vi "ViewEye.vi"(5 "new file path":path) -> ()   [LabVIEW 2022 SP3]
uses:
  -ReadEye/ScaleMethod.ctl
  <vilib>/Utility/miscctls.llb/LVPointDoubleTypeDef.ctl
  <vilib>/Utility/miscctls.llb/LVRectTypeDef.ctl
  <vilib>/Utility/miscctls.llb/LVOffsetAndMultiplierTypeDef.ctl
  <vilib>/Utility/miscctls.llb/LVBoundsTypeDef.ctl
  <vilib>/Analysis/baseanly.llb/Mean (DBL).vi
  <vilib>/Analysis/5stat.llb/RMS (DBL).vi
  <vilib>/Analysis/4window.llb/Chebyshev Window (DBL).vi
  <vilib>/Analysis/2dsp.llb/Zero Padder (DBL).vi
  <vilib>/Utility/file.llb/Write Delimited Spreadsheet (DBL).vi
  <vilib>/Utility/file.llb/Write Delimited Spreadsheet (string).vi
  <vilib>/Utility/file.llb/Read Delimited Spreadsheet (I64).vi
  <vilib>/Analysis/NI_AALPro.lvlib
  <vilib>/Analysis/NI_AALBase.lvlib
  <vilib>/ptbypt/NI_PtbyPt.lvlib
  <vilib>/gmath/NI_Gmath.lvlib
  <vilib>/Analysis/NI_AAL_SigProc.lvlib
panel:
  in  "Ref data":path=path "C:/WINDOWS/DESKTOP/rri.eye"
  in  "y":dbl(slide) scale=-2.0..2.0
  in  "RMS Save":bool
  in  "Boolean":bool
  in  "Flip Y":bool
  in  "Flip X":bool
  in  "Fill":bool
  in  "1-to-1":bool
  out "File Name":string
  in  "previously\nscanned":string
  in  "Keeper?":bool
  out "Scan Info":T1
  in  "File Ext":string="*.eye"
  out "Sound Speed":i16=1485
  in  "One Way":bool
  in  "Prev File":bool
  in  "Scale":bool=TRUE
  in  "Type of Mean":u16(ring) items=["Mean from lines", "Mean just lines", "Poly Mean", "No mean", "Filter"]
  in  "Filter Prams":T2={"low cutoff"=5, "order"=81, "high cutoff"=65}
  out "Raw data":dbl[][](graph)
  in  "Retro Parse":bool
  in  "Avg Spec":bool
  in  "Tab Control":T3(tab)
  in  "dB scale":u16(ring)=1 items=["Absolute", "Zero Ref"]
  in  "Vert Scale":u16(ring)=1 items=["Binary", "Dig Voltage", "Abs Voltage", "RF File Att Pram"]
  in  "Save RF":bool
  out "Blow up of blue Line":dbl[][](graph)
  out "Spectrum":T4(graph)
  in  "FFT size for":u16(ring)=9 items=["next 2^n", "8", "16", "32", "64", "128", "256", "512", "1024", "2048", "4096", "8192", "16384"]
  in  "Save Spectra?":bool
  out "blue win":dbl[](array[numeric])
  in  "Fit band":T5 {"center freq" format="%.2f"; "stop freq" format="%.2f"; "start" format="%.2f"}
  out "max doppler velocity mm/s":dbl
  in  "Drop freq coumn?":bool
  in  "Slide":cluster{dbl, dbl}(slide)={0.0, -50.63291139240506} scale=-80.0..100.0
  out "dB":dbl[][](graph)
  in  "STFT size":u16(ring)=9 items=["next 2^n", "8", "16", "32", "64", "128", "256", "512", "1024", "2048", "4096", "8192", "16384"]
  in  "Window":u32(ring)=2 items=["Rectangle"=0, "Hanning"=1, "Hamming"=2, "Blackman-Harris"=3, "Exact Blackman"=4, "Blackman"=5, "Flat Top"=6, "4 Term B-Harris "=7, "7 Term B-Harris"=8, "Low Sidelobe"=9, "Blackman Nuttall"=11, "Triangle"=30, "Gaussian"=62]
  out "mean 2":dbl format="%0.2f"
  out "mean":dbl format="%0.2f"
  out "Waveform Graph 2":dbl[](graph)
  out "Waveform Graph":dbl[](graph)
  in  "Spectro BMP":bool
  in  "Shift":sgl
  out "max value":sgl
  out "Time step (mics)":dbl
  in  "Spectrum?":bool
  out "Spectro fig":dbl[][](graph)
  in  "step size":i32=4 min=0
  in  "window pts":i32=64 min=0
  in  "Save Chirp":bool
  out "Match Data":dbl[][](graph)
  out "Chirp Temp":dbl[][](array[numeric])
  in  "Match Filter":bool
  in  "Add Lines":u16=1
  out "Axis scaling Params":T6 {"Y high" format="%.2f"; "Y low" format="%.2f"; "X left" format="%.2f"; "X right" format="%.2f"}
  out "inc y (mm)":dbl format="%.3f"
  out "inc x (mm)":dbl format="%.3f"
  in  "Reduce x data factor":i32=1
  in  "Pixels in y":i16=2500
  in  "Pixels in x":i16=256
  in  "Save BMP?":bool
  in  "Create Sector":bool
  out "Sector as data array":dbl[][](graph)
  out "cursor":dbl
  in  "Smooth factor":i32=1
  out "XY Graph":T7(graph)
  in  "Histo":bool
  in  "sub thresh":dbl=25.0
  in  "Contrast Batch":bool
  out "Therapy amplitude (mV)":sgl min=50 max=1000 format="%.2f"
  out "time trace":dbl[][](graph)
  out "Sepctra":cluster{i32, "df":dbl, dbl[][]}(graph)
  in  "Contrast Spec":bool
  out "Hit frac":dbl
  out "?":cluster{dbl[], "Best Linear Fit":dbl[]}[](graph)
  out "histogram":T7(graph)
  in  "Center Line SNR":bool
  out "Peaks":dbl[](graph)
  in  "save lateral?":bool
  out "Wire Locations RF pts":dbl[](array[numeric]) format="%0.2f"
  in  "Lateral beam":bool
  out "Wire Locations mm":dbl[](array[numeric]) format="%0.2f"
  out "lat beams":dbl[][](graph)
  in  "Threshold":i32=5000
  in  "width":i32=10
  out "SNRs":dbl[](array[numeric])
  in  "Wires":i32=13
  in  "Center index":i32
  out "Scan Line Peak":dbl[](array[numeric]) format="%0.2f"
  out "Beamwidths":sgl[](array[numeric])
  in  "initial Skip index":i32=100
  in  "Heart Trig":bool
  out "Smooth dat":dbl(graph)
  out "Avg Env image":dbl[][](graph)
  out "Overlay":dbl[][](graph)
  in  "AS Med Fil":i32=20
  in  "Edge Thresh":i32=20
  in  "Thresh Median Lngth":i32=10
  in  "direction":enum16{"either", "minus-plus", "plus-minus"}(ring)=enum."minus-plus"
  in  "neg cross":dbl=-3.0
  in  "Ebedded EKG":bool
  out "EKG":i16[][](graph)
  in  "EKG Gate":u16(ring) items=["Retro EKG", "Retro IQ"]
  out "dB 2":dbl[][](graph)
  out "Raw data 2":dbl[][](graph)
  in  "medians":i32=-1
  in  "left rank":i32=2
  in  "Log noise window":bool
  in  "Log":bool
  in  "CNR?":bool
  in  "Save RMS":bool
  out "Waveform Graph 3":dbl[](graph)
  in  "Save RF in window":bool
  in  "row to show":i32
  out "RMS dB BG":dbl format="%#.3g"
  out "CNR":dbl
  out "RMS flow dB":dbl format="%#.3g"
  out "dB CBR":dbl format="%#.3g"
  out "Spectrum 2":dbl[][](graph)
  out "RMS noise dB":dbl format="%#.3g"
  out "pk dB":dbl format="%#.2f"
  out "Pts  flow":i32
  out "Pts BG":i32
  out "Values":T8
  in  "ROI (mm)":T9={"X"=10.0, "Y"=10.0}
  in  "Fix Window CNR":bool
  in  "Delete File":bool
  in  "Whole Image":bool
  in  "Syn Focus":bool
  in  "Eye to BMP":bool
  in  "View Pics":bool
  in  "Alter Header":bool
  in  "Next File in Dir?":bool
  out "RF Lines":i32
  out "RF Window Pts":i32
  in  "ExitSendCmd":bool
  in  "Display mode":T10=enum."Log Grey Scale"
  out "DynRange":dbl format="%#.2f"
  out "RMS noise":dbl format="%#.3g"
  in  "Add Switch Noise?":bool
  in  "Axis scaling":bool
  in  "View Header?":bool
  in  "Header format":u16(ring) items=["Riverside Format", "Ron Linear", "GE Bin"]
  # "© 2000-2013 Riverside Research Institute"
  # "Ignore if not using a sector scan"
  # "Character to add to header"
  # "Note columns of the raw data have been inverted\nand the resulting matrix has been transposed to form\nthe sector image. Data reduced from raw form"
  # "Crop sides with yellow line"
  # "Use mm scale."
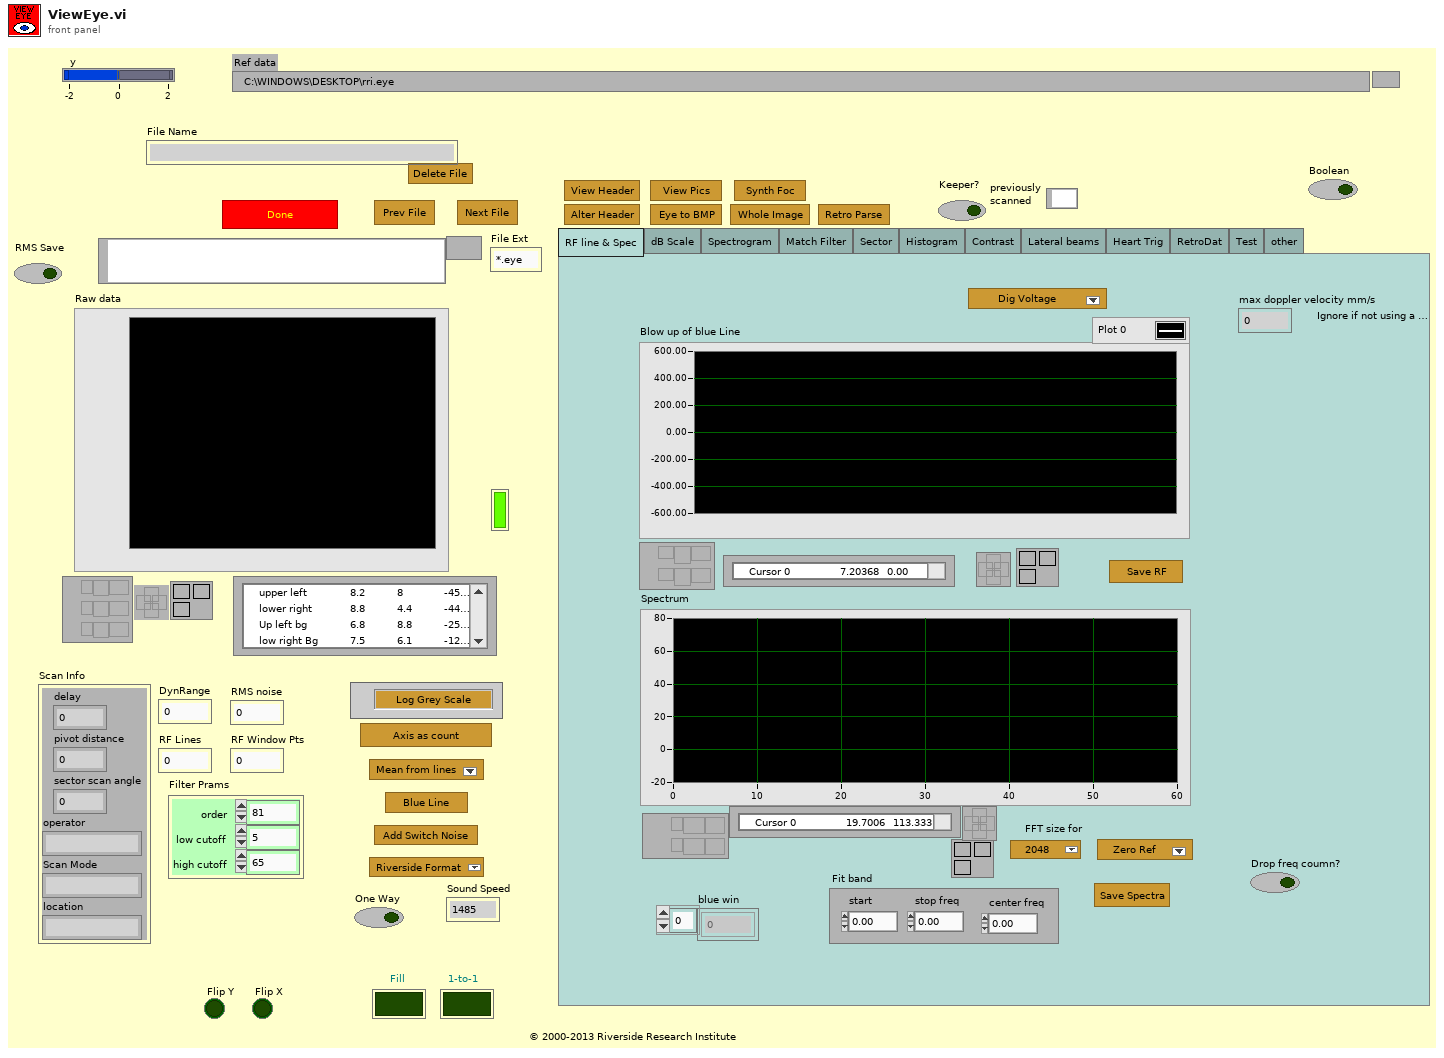
[diagram p1: front panel]
types:
  T1 = cluster{"delay":sgl, "pivot distance":sgl, "sector scan angle":sgl, "operator":string, "Scan Mode":string, "location":string}
  T2 = cluster{"low cutoff":i32, "order":i32, "high cutoff":i32}
  T3 = enum32{"RF line & Spec", "dB Scale", "Spectrogram", "Match Filter", "Sector", "Histogram", "Contrast", "Lateral beams", "Heart Trig", "RetroDat", "Test", "other"}
  T4 = cluster{"fo of fit":dbl, "df (MHz)":dbl, "Best Linear Fit":dbl[]}[]
  T5 = cluster{"start":dbl, "stop freq":dbl, "center freq":dbl}
  T6 = cluster{"X right":dbl, "X left":dbl, "Y low":dbl, "Y high":dbl}
  T7 = cluster{"X Values":dbl[], "Histogram: h(x)":i32[]}
  T8 = cluster{"mean":dbl, "variance":dbl, "mean":dbl, "variance":dbl}
  T9 = typedef "LVPointDoubleTypeDef.ctl" = cluster{"X":dbl, "Y":dbl}
  T10 = typedef "ScaleMethod.ctl" = enum16{"Linear Abs Grey", "Log Grey Scale", "Linear Color Scale", "dB Scale", "Verasonics Doppler"}
  T11 = typedef "LVRectTypeDef.ctl" = cluster{"Left":i16, "Top":i16, "Right":i16, "Bottom":i16}
  T12 = typedef "LVBoundsTypeDef.ctl" = cluster{"Width":u32, "Height":u32}
  T13 = cluster{"header info":cluster{"Header":string, "Head length":i16}, "A/D info":cluster{"# rf points per line":u16, "# lines per scan":u16, "sample rate MHz":u16, "# A/D bits":i16, "# bytes per A/D":u16, "TGC Flag":u16, "A/D Type":string}, "Tranducer Info":cluster{"bandwidth":sgl, "center freq":sgl, "start freq":sgl, "ID":i32}, "Scan Info":cluster{"delay":sgl, "pivot distance":sgl, "sector scan angle":sgl, "operator":string, "Scan Mode":string, "location":string}, "Time/Date Info":cluster{"date":string, "time":string}, "RF Info":cluster{"RF file name":string, "RF file att":string, "RF cal file name":string, "RF cal file att":string}, "Patient Info":cluster{"ID":string, "extended ID":string, "age":u16, "sex":string, "previously\nscanned":string, "PSA":sgl, "LOS":u8, "Ethnicty 2":u8, "Race":u8}, "Tissue Type":cluster{"organ":i16, "disease type":i16, "disease location":i16, "IQ_pts":u16, "RcvBuffer":u8, "RcvFrame":i16, "IQBuff":u8, "IQFrame":u16, "IQPage":u8}, "Votage scaling":cluster{"Digitizer (dB)":sgl, "Gain (dB)":sgl, "Atten (dB)":sgl}, "Comment":string, "Misc Items":cluster{"avg num":i16, "c speed":i16, "DivideBy":i16, "XMIT CHS":u8, "RCV CHS":u8, "Tx angle":u8}, "Therapy Parameters":cluster{"Theraputic Freq (MHz)":sgl, "Time on (s)":sgl, "Therapy amplitude (mV)":sgl, "Lines Before":u16, "Lines After":u16}, "Scan Settings":cluster{"Energy (microJ)":u8, "Damping (In Ohm)":u8, "HP Filt(KHz) ":u8, "LP Filt (MHz)":u8, "Gain (db)":u8, "prf (kHz)":sgl, "Distance between\nscan lines (mm)":u16, "Distance between\nscan planes (mm)":u16, "prf (kHz) 2":sgl, "prf (kHz) 3":sgl}, "Compression Parameters":cluster{"F1 (MHz)":sgl, "F2 (MHz)":sgl, "% taper":sgl, "duration":sgl}, "Patient Info Xtra":cluster{"First Name":string, "Last Name":string, "Notes":string}, "Boolean1":cluster{bool, bool, bool, bool, bool, bool, bool, bool, bool, bool, bool, bool, bool, bool, bool, bool, bool, bool, bool, bool, bool, bool}, "Boolean2":cluster{bool, bool, bool, bool, bool, bool, bool, bool, bool, bool, bool, bool, bool, bool, bool, bool, bool, bool, bool, bool, bool, bool, bool, bool, bool, bool, bool, bool, bool, bool, bool, bool, bool, bool, bool}, "Boolean3":cluster{bool, bool, bool, bool, bool, bool, bool, bool, bool, bool, bool, bool, bool, bool, bool, bool, bool, bool, bool, bool, bool, bool}}
  T14 = cluster{bool, bool, bool, bool, bool, bool, bool, bool, bool, bool, bool, bool, bool, bool, bool, bool, bool, bool, bool, bool, bool, bool}
  T15 = cluster{bool, bool, bool, bool, bool, bool, bool, bool, bool, bool, bool, bool, bool, bool, bool, bool, bool, bool, bool, bool, bool, bool, bool, bool, bool, bool, bool, bool, bool, bool, bool, bool, bool, bool, bool}
  T16 = enum16{"big-endian, network order", "native, host order", "little-endian"}
  T17 = typedef "Header.ctl" = cluster{"header info":cluster{"Header":string, "Head length":i16}, "A/D info":cluster{"# rf points per line":u16, "# lines per scan":u16, "sample rate MHz":u16, "# A/D bits":i16, "# bytes per A/D":u16, "TGC Flag":u16, "A/D Type":string}, "Tranducer Info":cluster{"bandwidth":sgl, "center freq":sgl, "start freq":sgl, "ID":i32}, "Scan Info":cluster{"delay":sgl, "pivot distance":sgl, "sector scan angle":sgl, "operator":string, "Scan Mode":string, "location":string}, "Time/Date Info":cluster{"date":string, "time":string}, "RF Info":cluster{"RF file name":string, "RF file att":string, "RF cal file name":string, "RF cal file att":string}, "Patient Info":cluster{"ID":string, "extended ID":string, "age":u16, "sex":string, "previously\nscanned":string, "PSA":sgl, "LOS":u8, "Ethnicty 2":u8, "Race":u8}, "Tissue Type":cluster{"organ":i16, "disease type":i16, "disease location":i16, "IQ_pts":u16, "RcvBuffer":u8, "RcvFrame":u16, "IQBuff":u8, "IQFrame":u16, "IQPage":u8}, "Votage scaling":cluster{"Digitizer (dB)":sgl, "Gain (dB)":sgl, "Atten (dB)":sgl}, "Comment":string, "Misc Info":cluster{"avg num":u16, "c speed":i16, "Div By or SF zones":i16, "XMIT CHS":u8, "RCV CHS":u8, "Xmit angle":sgl}, "Therapy Parameters":cluster{"Theraputic Freq (MHz)":sgl, "Time on (s)":sgl, "Therapy amplitude (mV)":sgl, "Lines Before":u16, "Lines After":u16}, "Scan Settings":cluster{"Energy (uJ or V)":u8, "Damp (Ohm) or Fc":u8, "HP Filt (KHz)":u8, "LP Filt (MHz)":u8, "Gain (db)":u8, "prf (kHz)":sgl, "Distance between\nscan lines (um)":u16, "Distance between\nscan planes (um)":u16, "Scan line gap (um)":sgl, "Scan plane gap (um)":sgl}, "Compression Parameters":cluster{"F1 (MHz)":sgl, "F2 (MHz)":sgl, "% taper":sgl, "duration":sgl}, "Patient Info Xtra":cluster{"First Name":string, "Last Name":string, "Notes":string}, "ROI Box":u16[]}
  T18 = cluster{"fo of fit":dbl, "df (MHz)":dbl, "Best Linear Fit":dbl[]}
  T19 = typedef "LVOffsetAndMultiplierTypeDef.ctl" = cluster{"Offset":dbl, "Multiplier":dbl}
  T20 = typedef "imagedata.ctl" = cluster{"image type":i32, "image depth":i32, "image":u8[], "mask":u8[], "colors":u32[], "Rectangle":cluster{"left":i16, "top":i16, "right":i16, "bottom":i16}}
  T21 = typedef "eventvkey.ctl" = enum16{"ASCII", "Enter", "Return", "Shift", "Ctrl", "Alt", "Cmd", "Opt", "Caps", "NumLock", "Clear", "Break", "Up", "Down", "Left", "Right", "Insert", "Delete", "Home", "End", "PageUp", "PageDown", "Escape", "Help", "Pause", "ScrollLock", "F1", "F2", "F3", "F4", "F5", "F6", "F7", "F8", "F9", "F10", "F11", "F12", "F13", "F14", "F15", "F16", "F17", "F18", "F19", "F20", "F21", "F22", "F23", "F24", "Play", "VolumeUp", "VolumeDown", "Mute", "Two Byte Char"}
  T22 = cluster{"Energy (microJ)":u8, "Damping (In Ohm)":u8, "HP Filt(KHz) ":u8, "LP Filt (MHz)":u8, "Gain (db)":u8, "prf (kHz)":sgl, "Distance between\nscan lines (um)":u16, "Distance between\nscan planes (um)":u16, "Scan line gap (um)":sgl, "Scan plane gap (um)":sgl}
  T23 = cluster{"Energy (uJ or V)":u8, "Damp (Ohm) or Fc":u8, "HP Filt (KHz)":u8, "LP Filt (MHz)":u8, "Gain (db)":u8, "prf (kHz)":sgl, "Distance between\nscan lines (um)":u16, "Distance between\nscan planes (um)":u16, "Scan line gap (um)":sgl, "Scan plane gap (um)":sgl}
  T24 = cluster{"# rf points per line":u16, "# lines per scan":u16, "sample rate MHz":u16, "# A/D bits":i16, "# bytes per A/D":u16, "TGC Flag":u16, "A/D Type":string}
  T25 = cluster{"bandwidth":sgl, "center freq":sgl, "start freq":sgl, "ID":i32}
  T26 = cluster{"RF file name":string, "RF file att":string, "RF cal file name":string, "RF cal file att":string}
  T27 = cluster{"ID":string, "extended ID":string, "age":u16, "sex":string, "previously\nscanned":string, "PSA":sgl, "LOS":u8, "Ethnicty 2":u8, "Race":u8}
  T28 = cluster{"organ":i16, "disease type":i16, "disease location":i16, "IQ_pts":u16, "RcvBuffer":u8, "RcvFrame":u16, "IQBuff":u8, "IQFrame":u16, "IQPage":u8}
  T29 = cluster{"Digitizer (dB)":sgl, "Gain (dB)":sgl, "Atten (dB)":sgl}
  T30 = cluster{"avg num":u16, "c speed":i16, "Div By or SF zones":i16, "XMIT CHS":u8, "RCV CHS":u8, "Xmit angle":sgl}
  T31 = cluster{"Theraputic Freq (MHz)":sgl, "Time on (s)":sgl, "Therapy amplitude (mV)":sgl, "Lines Before":u16, "Lines After":u16}
  T32 = cluster{"F1 (MHz)":sgl, "F2 (MHz)":sgl, "% taper":sgl, "duration":sgl}
  T33 = cluster{"First Name":string, "Last Name":string, "Notes":string}
  T34 = cluster{"max f":sgl, "max freq (dB)":sgl, "center freq":sgl, "lower band freq":sgl, "upper band freq":sgl, "bandwidth":sgl, "% BW":dbl}
  T35 = cluster{"40 MHz mean":dbl, "40 MHz SD":dbl, "Ratio Mean":dbl, "Ratio SD":dbl, "Hit frac":dbl, "Hit Num":i32, "slope cum":dbl, "r^2 cum":dbl, "slope sub":dbl, "r^2 sub":dbl}
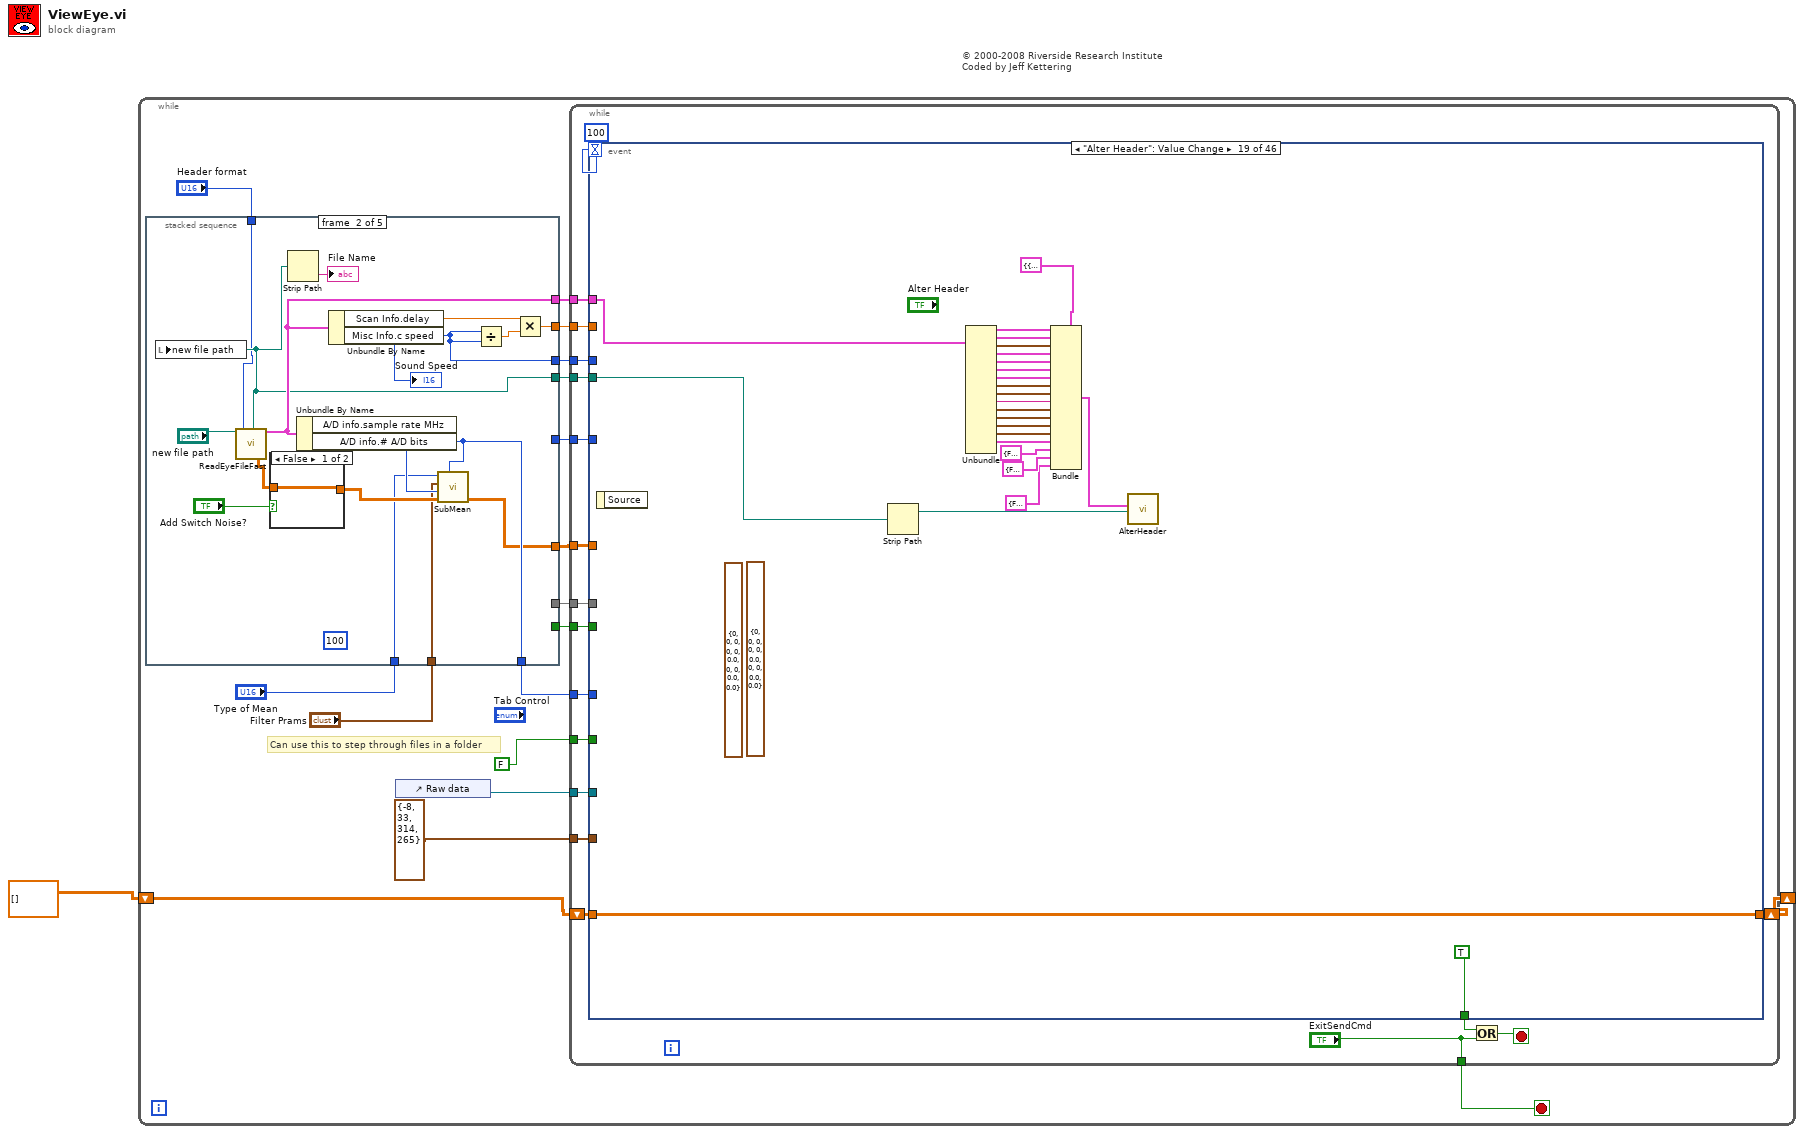
[diagram p0: block diagram]
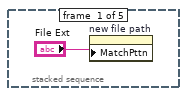
[diagram p2: hidden frame]
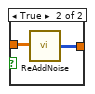
[diagram p3: hidden frame]
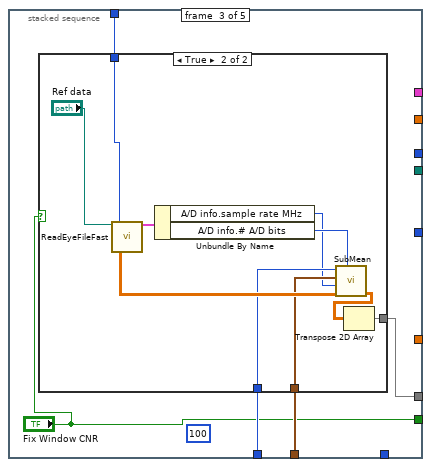
[diagram p4: hidden frame]
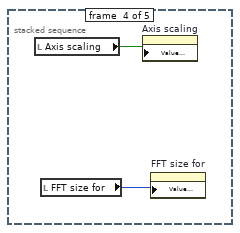
[diagram p6: hidden frame]
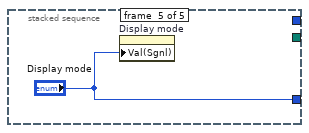
[diagram p7: hidden frame]
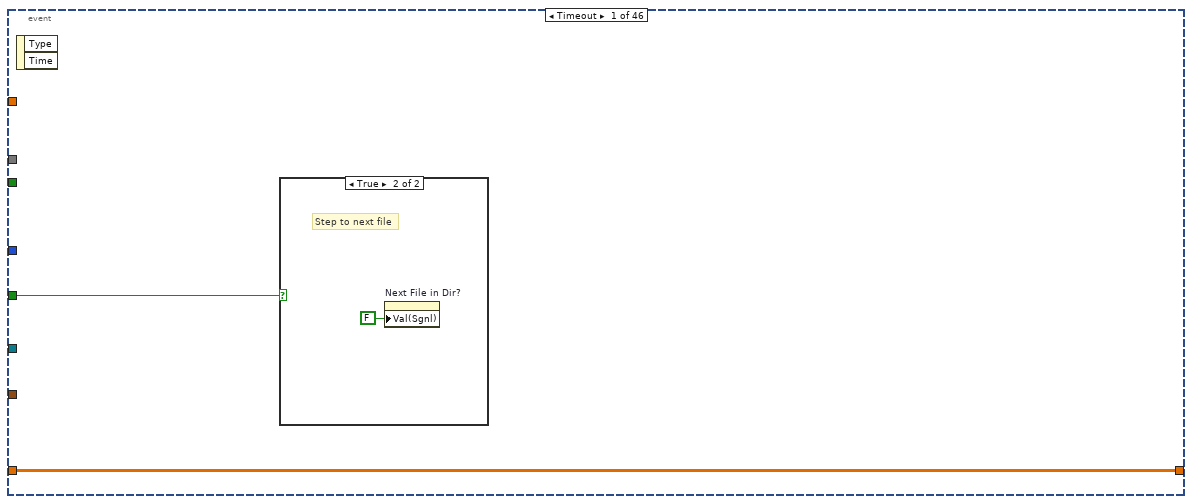
[diagram p8: hidden frame]
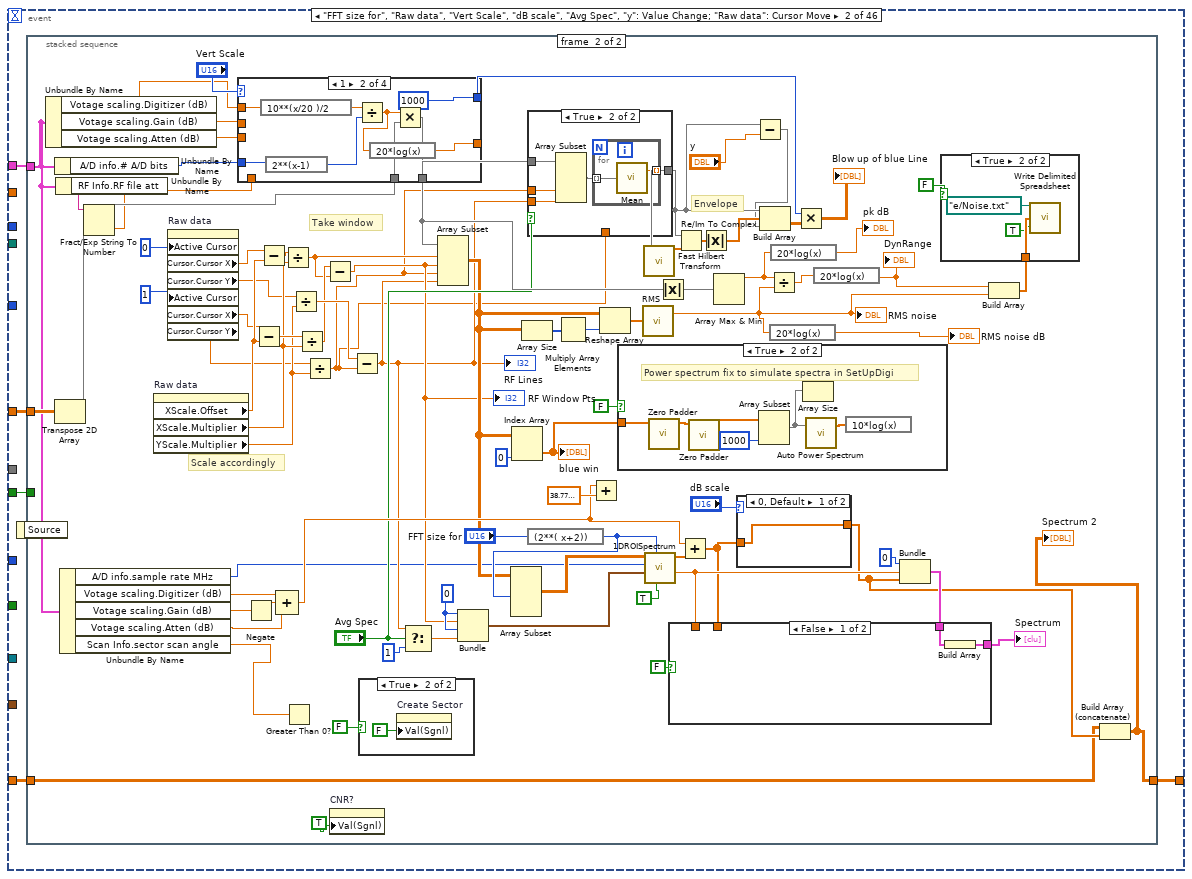
[diagram p10: hidden frame]
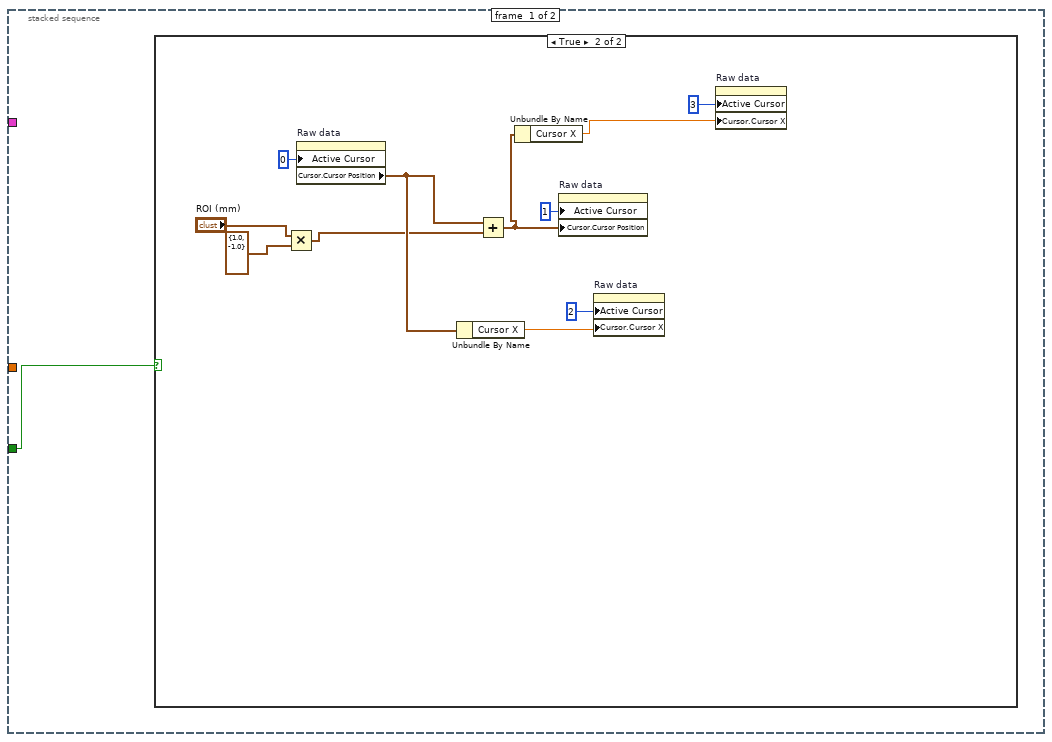
[diagram p11: hidden frame]
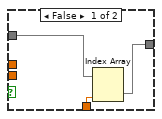
[diagram p13: hidden frame]
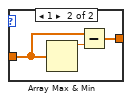
[diagram p17: hidden frame]
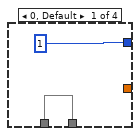
[diagram p18: hidden frame]
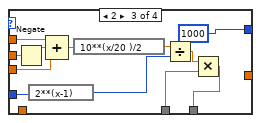
[diagram p19: hidden frame]
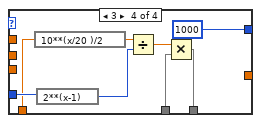
[diagram p20: hidden frame]
diagram:
  # "© 2000-2008 Riverside Research Institute\nCoded by Jeff Kettering"
  n1 = while {
    shift-right: [w8] -> _
    shift-left: dbl[][] [] -> [w7]
    stop <- w18 stop-if-true
    # "Can use this to step through files in a folder"
    n2 = stacked-sequence {
      tunnel: [_ w24 _ _ _] -> w19
      tunnel: [_ w30 _ _ _] -> w17
      tunnel: [_ _ _ _ "Display mode"] -> w16
      tunnel: [_ w31 _ _ _] -> w15
      tunnel: [_ w33 _ _ _] -> w14
      tunnel: [_ w28 _ _ _] -> w13
      tunnel: [_ w27 _ _ _] -> w9
      tunnel: "Filter Prams" -> [_ w23 w45 _ _]
      tunnel: "Type of Mean" -> [_ w22 w44 _ _]
      tunnel: "Header format" -> [_ w21 w43 _ _]
      tunnel: [_ _ w42 _ _] -> w3
      tunnel: [_ _ "Fix Window CNR" _ _] -> w2
      frame #0 {
        n3 = property on="new file path" class="Path"("MatchPttn"="File Ext") -> ()  [unwired: 2 in, 2 out]
      }
      frame #1 {
        (unwired) 100 ("y")
        n4 = call "ReadEyeFileFast.vi"("new file path"="new file path", "Header format"=w21) -> ("new path out"=w30:path, "2-D data array"=w26:sgl[][], "Header In"=w31:T17)  [unwired: 15 out]
        n5 = local write "new file path"(w30) -> ()
        n6 = case shown="False" "Add Switch Noise?" {
          tunnel: w26 -> [w38 w40]
          tunnel: [w38 w39] -> w25
          frame False {
          }
          frame True {
            n7 = call "ReAddNoise.vi"("Data in"=w40) -> ("Data out"=w39:i16[][])
          }
        }
        n8 = Strip Path(path=w30) -> (name=→"File Name":string)  [unwired: 1 out]
        n9 = Unbundle By Name(w31) -> ("A/D info.sample rate MHz"=w32:u16, "A/D info.# A/D bits"=w27:i16)
        n10 = Unbundle By Name(w31) -> ("Scan Info.delay"=w34:sgl, "Misc Info.c speed"=w28:i16)
        "Sound Speed" <- w28
        n11 = call "SubMean.vi"("Bit Depth"=w27, "Scan Data In"=w25, "Samp Rate (MHz)"=w32, "Filter Prams"=w23, "Type of Mean"=w22) -> ("Array"=w24:dbl[][])  [unwired: 1 in, 2 out]
        n12 = Divide(x=w28, y=w28) -> (x/y=w35:dbl)
        n13 = Multiply(x=w34, y=w35) -> (x*y=w33:dbl)
      }
      frame #2 {
        (unwired) 100 ("y")
        n14 = case shown="True" "Fix Window CNR" {
          tunnel: w45 -> [_ w54]
          tunnel: w44 -> [_ w53]
          tunnel: w43 -> [_ w49]
          tunnel: [_ w46] -> w42
          frame False {
          }
          frame True {
            n15 = call "ReadEyeFileFast.vi"("new file path"="Ref data", "Header format"=w49) -> ("2-D data array"=w55:sgl[][], "Header In"=w52:T17)  [unwired: 16 out]
            n16 = Unbundle By Name(w52) -> ("A/D info.sample rate MHz"=w50:u16, "A/D info.# A/D bits"=w51:i16)
            n17 = call "SubMean.vi"("Bit Depth"=w51, "Scan Data In"=w55, "Samp Rate (MHz)"=w50, "Filter Prams"=w54, "Type of Mean"=w53) -> ("Array"=w47:dbl[][])  [unwired: 1 in, 2 out]
            n18 = Transpose 2D Array(2D array=w47) -> (transposed array=w46:dbl[][])
          }
        }
      }
      frame #3 {
        n19 = local read "Axis scaling"() -> (w56:bool)
        n20 = local read "FFT size for"() -> (w57:u16)
        n21 = property on="Axis scaling" class="Bool (strict)"("Value (Signaling)"=w56) -> ()  [unwired: 2 in, 2 out]
        n22 = property on="FFT size for" class="Ring (strict)"("Value (Signaling)"=w57) -> ()  [unwired: 2 in, 2 out]
      }
      frame #4 {
        n23 = property on="Display mode" class="Enum (strict)"("Val(Sgnl)"="Display mode") -> ()  [unwired: 2 in, 2 out]
      }
    }
    n24 = control-ref of="Raw data"() -> (w11:refnum<vi>)
    n25 = while {
      tunnel: w19 -> [w76]
      tunnel: w17 -> [w74]
      tunnel: w16 -> [w73]
      tunnel: ["ExitSendCmd"] -> w18
      tunnel: w15 -> [w69]
      tunnel: w14 -> [w68]
      tunnel: w13 -> [w67]
      tunnel: FALSE -> [w66]
      tunnel: T11 {"Left"=-8, "Top"=33, "Right"=314, "Bottom"=265} ("Plot Area Bounds") -> [w65]
      tunnel: w11 -> [w64]
      tunnel: w9 -> [w63]
      shift-right: [w62] -> w8
      shift-left: w7 -> [w61]
      tunnel: w3 -> [w60]
      tunnel: w2 -> [w59]
      stop <- w70 stop-if-true
      n26 = event shown="[18] \"Alter Header\": Value Change" {
        selector: _ -> [_ _ _ _ _ _ _ _ _ _ _ _ _ _ _ _ _ _ _ _ _ _ _ _ _ _ _ _ _ _ _ _ _ _ _ _ _ _ _ _ _ _ _ _ _ _]
        dyn-events: _ -> [_ _ _ _ _ _ _ _ _ _ _ _ _ _ _ _ _ _ _ _ _ _ _ _ _ _ _ _ _ _ _ _ _ _ _ _ _ _ _ _ _ _ _ _ _ _]
        timeout: 100 -> [_ _ _ _ _ _ _ _ _ _ _ _ _ _ _ _ _ _ _ _ _ _ _ _ _ _ _ _ _ _ _ _ _ _ _ _ _ _ _ _ _ _ _ _ _ _]
        tunnel: w76 -> [_ w84 _ w338 w396 _ w491 _ _ _ w595 _ _ _ _ _ _ _ _ _ _ _ _ _ _ _ _ _ w890 w984 _ _ _ w1059 _ w1085 _ _ w1109 _ _ _ _ _ _ _]
        tunnel: w74 -> [_ _ _ w317 w409 w489 w503 _ _ _ _ _ w669 w692 w713 _ w751 _ w789 _ _ _ _ w844 _ w849 w852 w855 w861 _ _ _ w1045 _ w1069 _ w1095 w1106 _ w1176 _ _ w1229 _ _ w1244]
        tunnel: w73 -> [_ _ _ _ _ _ _ _ _ _ _ _ _ _ _ _ _ _ _ _ _ _ _ _ _ _ _ _ _ _ _ _ _ _ _ _ _ _ _ _ _ _ _ _ _ _]
        tunnel: [_ _ _ _ _ _ _ _ _ _ _ TRUE _ _ TRUE _ TRUE TRUE TRUE _ _ _ _ _ TRUE _ _ _ _ _ _ _ _ _ _ _ _ _ _ _ TRUE TRUE TRUE TRUE TRUE TRUE] -> w71
        tunnel: w69 -> [_ w83 _ w327 w417 _ w493 _ w541 _ w608 _ w659 w699 _ _ _ _ w786 w792 _ _ _ _ _ _ _ _ w878 _ w999 _ _ w1056 _ w1071 w1099 _ _ w1173 _ _ w1232 _ _ w1246]
        tunnel: w68 -> [_ _ _ _ _ _ _ _ _ _ _ _ _ _ _ _ _ _ _ _ _ _ _ _ _ _ _ _ w876 _ _ _ _ _ _ _ _ _ _ _ _ _ _ _ _ _]
        tunnel: w67 -> [_ _ _ _ _ _ _ _ w542 _ _ _ _ _ _ _ _ _ _ _ _ _ _ _ _ _ _ _ w877 _ _ _ _ _ _ _ _ _ _ _ _ _ _ _ _ _]
        tunnel: w66 -> [w78 _ _ _ _ _ w494 _ _ _ _ _ _ _ _ _ _ _ _ _ _ _ _ _ _ _ _ _ _ _ _ _ _ _ _ _ _ _ _ _ _ _ _ _ _ _]
        tunnel: w65 -> [_ _ _ _ _ _ _ _ _ _ _ _ _ _ _ _ _ _ _ w793 w835 _ _ _ _ _ _ _ _ _ _ _ _ _ _ _ _ _ _ _ _ _ _ _ _ _]
        tunnel: w64 -> [_ _ _ _ _ _ _ _ _ _ _ _ _ _ _ _ _ _ _ w791 _ w837 w840 _ _ _ _ _ _ _ _ _ _ _ _ _ _ _ _ _ _ _ _ _ _ _]
        tunnel: w63 -> [_ _ _ _ _ _ _ _ _ _ _ _ _ _ _ _ _ _ _ _ _ _ _ _ _ _ _ _ _ _ _ _ _ _ _ _ _ _ w1108 _ _ _ _ _ _ _]
        tunnel: [w77 w81 w251 w274 w392 w487 w492 w533 w537 w544 w568 w643 w647 w686 w709 w733 w741 w763 w766 w790 w834 w836 w839 w842 w845 w847 w850 w853 w871 w976 w997 w1036 w1039 w1055 w1067 w1070 w1087 w1104 w1107 w1172 w1216 w1218 w1220 w1233 w1235 w1237] -> w62
        tunnel: w61 -> [w77 w82 w251 w274 w392 w487 w492 w533 w537 w544 w568 w643 w647 w686 w709 w733 w741 w763 w766 w790 w834 w836 w839 w842 w845 w847 w850 w853 w871 w976 w997 w1036 w1039 w1055 w1067 w1070 w1087 w1104 w1107 w1172 w1216 w1218 w1220 w1233 w1235 w1237]
        tunnel: w60 -> [_ _ _ w263 _ _ _ _ _ _ _ _ _ _ _ _ _ _ _ _ _ _ _ _ _ _ _ _ _ _ _ _ _ _ _ _ _ _ _ _ _ _ _ _ _ _]
        tunnel: w59 -> [_ w80 _ _ _ _ _ _ _ _ _ _ _ _ _ _ _ _ _ _ _ _ _ _ _ _ _ _ _ _ _ _ _ _ _ _ _ _ _ _ _ _ _ _ _ _]
        event Timeout {
          n27 = event-data() -> ()  [unwired: 3 out]
          n28 = case shown="True" w78 {
            frame False {
            }
            frame True {
              # "Step to next file"
              n29 = property on="Next File in Dir?" class="Bool (strict)"("Val(Sgnl)"=FALSE ("Value (Signaling)")) -> ()  [unwired: 2 in, 2 out]
            }
          }
        }
        event "FFT size for", "Raw data", "Vert Scale", "dB scale", "Avg Spec", "y": Value Change; "Raw data": Cursor Move {
          n30 = event-data() -> ()  [unwired: 2 out]
          n31 = stacked-sequence {
            tunnel: w84 -> [_ w163]
            tunnel: w83 -> [_ w119]
            tunnel: w82 -> [_ w107]
            tunnel: [_ w106] -> w81
            tunnel: w80 -> [w85 _]
            frame #0 {
              n32 = case shown="True" w85 {
                frame False {
                }
                frame True {
                  n33 = Multiply(x="ROI (mm)", y=T9 {"X"=1.0, "Y"=-1.0}) -> (x*y=w86:T9)
                  n34 = property on="Raw data" class="IntGraph (strict)"("Active Cursor"=u32 0 ("Write Attribute")) -> ("Cursor.Cursor Position"=w93:T9)  [unwired: 2 in, 2 out]
                  n35 = Unbundle By Name(w93) -> ("Cursor X"=w92:dbl)
                  n36 = Add(x=w93, y=w86) -> (x+y=w88:T9)
                  n37 = Unbundle By Name(w88) -> ("Cursor X"=w90:dbl)
                  n38 = property on="Raw data" class="IntGraph (strict)"("Active Cursor"=u32 1 ("Write Attribute"), "Cursor.Cursor Position"=w88) -> ()  [unwired: 2 in, 2 out]
                  n39 = property on="Raw data" class="IntGraph (strict)"("Active Cursor"=u32 2 ("Write Attribute"), "Cursor.Cursor X"=w92) -> ()  [unwired: 2 in, 2 out]
                  n40 = property on="Raw data" class="IntGraph (strict)"("Active Cursor"=u32 3 ("Write Attribute"), "Cursor.Cursor X"=w90) -> ()  [unwired: 2 in, 2 out]
                }
              }
            }
            frame #1 {
              w148 = 0
              # "Envelope"
              # "Take window"
              # "Scale accordingly"
              n41 = Unbundle By Name(w119) -> ("Votage scaling.Digitizer (dB)"=w97:sgl, "Votage scaling.Gain (dB)"=w146:sgl, "Votage scaling.Atten (dB)"=w144:sgl)
              n42 = Unbundle By Name(w119) -> ("A/D info.# A/D bits"=w145:i16)
              n43 = Transpose 2D Array(2D array=w163) -> (transposed array=w128:dbl[][])
              n44 = Unbundle By Name(w119) -> ("RF Info.RF file att"=w160:string)
              n45 = Unbundle By Name(w119) -> ("A/D info.sample rate MHz"=w111:u16, "Votage scaling.Digitizer (dB)"=w123:sgl, "Votage scaling.Gain (dB)"=w124:sgl, "Votage scaling.Atten (dB)"=w125:sgl, "Scan Info.sector scan angle"=w120:sgl)
              n46 = Fract/Exp String To Number(string=w160) -> (number=w122:dbl)  [unwired: 4 out]
              n47 = property on="Raw data" class="IntGraph (strict)"() -> ("XScale.Offset"=w159:dbl, "XScale.Multiplier"=w158:dbl, "YScale.Multiplier"=w157:dbl)  [unwired: 2 in, 2 out]
              n48 = property on="Raw data" class="IntGraph (strict)"("Active Cursor"=u32 0 ("Write Attribute"), "Active Cursor"=u32 1 ("Write Attribute")) -> ("Cursor.Cursor X"=w156:dbl, "Cursor.Cursor Y"=w152:dbl, "Cursor.Cursor X"=w155:dbl, "Cursor.Cursor Y"=w151:dbl)  [unwired: 2 in, 2 out]
              n49 = case shown="1" "Vert Scale" {
                tunnel: w145 -> [_ w213 w221 w234]
                tunnel: w97 -> [_ w214 w226 _]
                tunnel: w144 -> [_ _ w225 _]
                tunnel: w146 -> [_ _ w223 _]
                tunnel: w128 -> [w205 w210 w217 w230]
                tunnel: [w205 w209 w216 w229] -> w117
                tunnel: w122 -> [_ _ _ w228]
                tunnel: [1 1000 1000 1000] -> w136
                tunnel: [_ w206 _ _] -> _
                frame 0, Default {
                }
                frame 1 {
                  n50 = expression code="10**(x/20 )/2"(w214) -> (w212:sgl)
                  n51 = expression code="2**(x-1)"(w213) -> (w211:i16)
                  n52 = Divide(x=w212, y=w211) -> (x/y=w207:sgl)
                  n53 = expression code="20*log(x)"(w207) -> (w206:sgl)
                  n54 = Multiply(x=w207, y=w210) -> (x*y=w209:dbl[][])
                }
                frame 2 {
                  n55 = Negate(x=w223) -> (-x=w224:sgl)
                  n56 = expression code="2**(x-1)"(w221) -> (w219:i16)
                  n57 = Compound Arithmetic op=ADD(w226, w224, w225) -> (w222:sgl)
                  n58 = expression code="10**(x/20 )/2"(w222) -> (w220:sgl)
                  n59 = Divide(x=w220, y=w219) -> (x/y=w218:sgl)
                  n60 = Multiply(x=w218, y=w217) -> (x*y=w216:dbl[][])
                }
                frame 3 {
                  n61 = expression code="10**(x/20 )/2"(w228) -> (w233:dbl)
                  n62 = expression code="2**(x-1)"(w234) -> (w232:i16)
                  n63 = Divide(x=w233, y=w232) -> (x/y=w231:dbl)
                  n64 = Multiply(x=w231, y=w230) -> (x*y=w229:dbl[][])
                }
              }
              n65 = Negate(x=w124) -> (-x=w126:sgl)
              n66 = Subtract(x=w155, y=w159) -> (x-y=w165:dbl)
              n67 = Subtract(x=w156, y=w159) -> (x-y=w166:dbl)
              n68 = Compound Arithmetic op=ADD(w123, w126, w125) -> (w121:sgl)
              n69 = Divide(x=w166, y=w158) -> (x/y=w150:dbl)
              n70 = Greater Than 0?(x=w120) -> ()  [unwired: 1 out]
              n71 = Divide(x=w152, y=w157) -> (x/y=w167:dbl)
              n72 = Divide(x=w165, y=w158) -> (x/y=w164:dbl)
              n73 = Divide(x=w151, y=w157) -> (x/y=w101:dbl)
              n74 = Subtract(x=w164, y=w150) -> (x-y=w114:dbl)
              "RF Window Pts" <- w114
              n75 = property on="CNR?" class="Bool (strict)"("Val(Sgnl)"=TRUE ("Value (Signaling)")) -> ()  [unwired: 2 in, 2 out]
              n76 = Subtract(x=w167, y=w101) -> (x-y=w112:dbl)
              "RF Lines" <- w112
              n77 = case shown="True" FALSE {
                frame False {
                }
                frame True {
                  n78 = property on="Create Sector" class="Bool (strict)"("Val(Sgnl)"=FALSE ("Value (Signaling)")) -> ()  [unwired: 2 in, 2 out]
                }
              }
              n79 = Select(t=w112, s="Avg Spec", f=1) -> (s? t:f=w113:dbl)
              n80 = Array Subset(array=w117, index (row)=w150, length (row)=w114, index (col)=w101, length (col)=w112) -> (w115:dbl[][])
              n81 = Bundle(w148, w114, w148, w113) -> (w174:cluster{i32, dbl, i32, dbl})  [unwired: 1 out]
              n82 = Index Array(array=w115, index (col)=0) -> (element=w140:dbl[])  [unwired: 1 in]
              "blue win" <- w140
              n83 = Array Size(array=w115) -> (size(s)=w176:i32[])
              n84 = case shown="True" "Avg Spec" {
                tunnel: w117 -> [w182 w185]
                tunnel: w101 -> [w181 _]
                tunnel: [w180 w186] -> w100
                tunnel: w112 -> [_ w184]
                tunnel: w101 -> [_ w183]
                frame False {
                  n85 = Index Array(array=w182, index (col)=w181) -> (element=w180:dbl[])  [unwired: 1 in]
                }
                frame True {
                  n86 = Array Subset(array=w185, index (col)=w183, length (col)=w184) -> (w187:dbl[][])  [unwired: 2 in]
                  n87 = for {
                    tunnel: w187 -> [w189] mode=indexing
                    tunnel: [w188] -> w186 mode=indexing
                    n88 = call-poly <vilib>:"Mean.vi"("X"=w189) -> ("mean"=w188:dbl)  [unwired: 1 out]
                  }
                }
              }
              n89 = expression code="(2**( x+2))"("FFT size for") -> (w129:u16)
              n90 = Array Subset(array=w115, length (row)=w129) -> (w130:dbl[][])  [unwired: 3 in]
              n91 = Multiply Array Elements(1:w176) -> (0:w175:i32)
              n92 = Add(x=w121, y=sgl 38.78) -> ()  [unwired: 1 out]
              n93 = Reshape Array(w115, w175) -> (w110:dbl[])
              n94 = case shown="True" FALSE {
                tunnel: w140 -> [_ w197]
                frame False {
                }
                frame True {
                  # "Power spectrum fix to simulate spectra in SetUpDigi"
                  n95 = call-poly <vilib>:"Zero Padder.vi"("Input Array"=w197) -> ("Zero Padded Array"=w199:dbl[])  [unwired: 10 in]
                  n96 = call-poly <vilib>:"Zero Padder.vi"("Input Array"=w199) -> ("Zero Padded Array"=w195:dbl[])  [unwired: 10 in]
                  n97 = Array Subset(array=w195, length=1000) -> (w194:dbl[])  [unwired: 1 in]
                  n98 = Array Size(array=w194) -> ()  [unwired: 1 out]
                  n99 = call <vilib>:"Auto Power Spectrum.vi"("Signal (V)"=w194) -> ("Power Spectrum (V^2 rms)"=w196:dbl[])  [unwired: 1 in, 1 out]
                  n100 = expression code="10*log(x)"(w196) -> ()  [unwired: 1 out]
                }
              }
              n101 = call-poly <vilib>:"RMS.vi"("X"=w110) -> ("rms value"=w105:dbl)  [unwired: 1 out]
              "RMS noise" <- w105
              n102 = call <vilib>:"Fast Hilbert Transform.vi"("X"=w100) -> ("Hilbert{X}"=w179:dbl[])  [unwired: 1 out]
              n103 = call "1DROISpectrum.vi"("convert output to dB?"=TRUE, "Length of padded array"=w129, "Array Subset"=w174, "freq (MHz)"=w111, "2-D data array"=w130) -> ("df (MHz)"=w171:dbl, "power spectrum in dB"=w161:dbl[])  [unwired: 5 out]
              n104 = Absolute Value(x=w117) -> (abs(x)=w133:dbl[][])
              n105 = Re/Im To Complex(1:w179, 2:w100) -> (0:w178:cdb[])
              n106 = Add(x=w121, y=w161) -> (x+y=w141:dbl[])
              n107 = Absolute Value(x=w178) -> (abs(x)=w177:dbl[])
              n108 = Array Max & Min(array=w133) -> (max value=w103:dbl)  [unwired: 3 out]
              n109 = case shown="0, Default" "dB scale" {
                tunnel: [w200 w203] -> w108
                tunnel: w141 -> [w200 w201]
                frame 0, Default {
                }
                frame 1 {
                  n110 = Array Max & Min(array=w201) -> (max value=w202:dbl)  [unwired: 3 out]
                  n111 = Subtract(x=w201, y=w202) -> (x-y=w203:dbl[])
                }
              }
              n112 = Subtract(x=w100, y="y") -> (x-y=w99:dbl[])
              n113 = Build Array(w100, w177, w99) -> (w137:dbl[][])
              n114 = Divide(x=w103, y=w105) -> (x/y=w131:dbl)
              n115 = expression code="20*log(x)"(w105) -> (→"RMS noise dB":dbl)
              n116 = expression code="20*log(x)"(w103) -> (→"pk dB":dbl)
              n117 = Multiply(x=w136, y=w137) -> (x*y=→"Blow up of blue Line":dbl[][])
              n118 = expression code="20*log(x)"(w131) -> (w132:dbl)
              "DynRange" <- w132
              n119 = Bundle(0, "df (MHz)"=w171, w108) -> (w169:cluster{i32, "df (MHz)":dbl, dbl[]})  [unwired: 1 out]
              n120 = case shown="False" FALSE ("Case Constant\n(See Context Help)") {
                tunnel: w171 -> [_ w241]
                tunnel: w141 -> [_ w240]
                tunnel: w169 -> [w236 w238]
                tunnel: [w235 w237] -> w168
                frame False {
                  n121 = Build Array(w236) -> (w235:cluster{i32, "df (MHz)":dbl, dbl[]}[])
                }
                frame True {
                  # "Find spectral fit"
                  n122 = call "FitSpectrum.vi"("Y Values"=w240, "df (MHz)"=w241, "Fit band"="Fit band") -> ("fo of fit"=w242:dbl, "Best Linear Fit"=w243:dbl[])  [unwired: 11 out]
                  n123 = Bundle("fo of fit"=w242, "df (MHz)"=w241, "Best Linear Fit"=w243) -> (w239:T18)  [unwired: 1 out]
                  n124 = Build Array(w238, w239) -> (w237:T4)
                }
              }
              "Spectrum" <- w168
              n125 = Build Array(w132, w105) -> (w135:dbl[])
              n126 = case shown="True" FALSE {
                tunnel: w135 -> [_ w193]
                frame False {
                }
                frame True {
                  n127 = call-poly <vilib>:"Write Delimited Spreadsheet.vi"("file path (dialog if empty)"=path "e:/Noise.txt", "1D data"=w193, "transpose? (no:F)"=TRUE ("append to file? (new file:F)")) -> ()  [unwired: 11 in, 2 out]
                }
              }
              n128 = Build Array (concatenate)(w107, w108) -> (w106:dbl[][])
              "Spectrum 2" <- w106
            }
          }
        }
        event "RMS Save": Value Change {
          n129 = event-data() -> ()  [unwired: 7 out]
          n130 = local read "RMS noise"() -> (w248:dbl)
          n131 = property on="Raw data" class="IntGraph (strict)"("Active Cursor"=u32 0) -> ("Cursor.Cursor X"=w249:dbl)  [unwired: 2 in, 2 out]
          n132 = Build Array(w249, w248) -> (w247:dbl[])
          n133 = call-poly <vilib>:"Write Delimited Spreadsheet.vi"("file path (dialog if empty)"=path "C:/Users/jketterling/Desktop/mp.txt", "1D data"=w247, "append to file? (new file:F)"=TRUE) -> ()  [unwired: 11 in, 2 out]
        }
        event "CNR?", "Save RMS": Value Change {
          # "RMS FLow\nRMS BG\ndB CBR\nCNR\nmean env flow\nvar flow\nmean env bg\nvar bg\nROI X dim\nROI Y dim\ndepth"
          # "Bflow/anechoic"
          # "Background"
          # "Take window"
          # "Scale accordingly"
          # "Take window"
          # "Scale accordingly"
          n134 = event-data() -> ()  [unwired: 7 out]
          n135 = Unbundle By Name(w327) -> ("RF Info.RF file att"=w337:string)
          n136 = Transpose 2D Array(2D array=w338) -> (transposed array=w330:dbl[][])
          n137 = Unbundle By Name(w327) -> ("Votage scaling.Digitizer (dB)"=w329:sgl, "Votage scaling.Gain (dB)"=w333:sgl, "Votage scaling.Atten (dB)"=w331:sgl)
          n138 = local read "Vert Scale"() -> (w315:u16)
          n139 = Unbundle By Name(w327) -> ("A/D info.# A/D bits"=w332:i16)
          n140 = Fract/Exp String To Number(string=w337) -> (number=w328:dbl)  [unwired: 4 out]
          n141 = property on="Raw data" class="IntGraph (strict)"() -> ("XScale.Offset"=w289:dbl, "XScale.Multiplier"=w288:dbl, "YScale.Multiplier"=w287:dbl)  [unwired: 2 in, 2 out]
          n142 = property on="Raw data" class="IntGraph (strict)"("Active Cursor"=u32 0 ("Write Attribute"), "Active Cursor"=u32 1 ("Write Attribute")) -> ("Cursor.Cursor X"=w255:dbl, "Cursor.Cursor Y"=w257:dbl, "Cursor.Cursor X"=w253:dbl, "Cursor.Cursor Y"=w259:dbl)  [unwired: 2 in, 2 out]
          n143 = property on="Raw data" class="IntGraph (strict)"("Active Cursor"=u32 2 ("Write Attribute"), "Active Cursor"=u32 3 ("Write Attribute")) -> ("Cursor.Cursor X"=w310:dbl, "Cursor.Cursor Y"=w306:dbl, "Cursor.Cursor X"=w309:dbl, "Cursor.Cursor Y"=w305:dbl)  [unwired: 2 in, 2 out]
          n144 = case shown="True" FALSE {
            frame False {
            }
            frame True {
              n145 = property on="Next File in Dir?" class="Bool (strict)"("Val(Sgnl)"=TRUE ("Value (Signaling)")) -> ()  [unwired: 2 in, 2 out]
            }
          }
          n146 = case shown="1" w315 {
            tunnel: w332 -> [_ w370 w378 w391]
            tunnel: w329 -> [_ w371 w383 _]
            tunnel: w331 -> [_ _ w382 _]
            tunnel: w333 -> [_ _ w380 _]
            tunnel: w330 -> [w363 w367 w374 w387]
            tunnel: [w363 w366 w373 w386] -> w264
            tunnel: w328 -> [_ _ _ w385]
            tunnel: [1 1000 1000 1000] -> w298
            frame 0, Default {
            }
            frame 1 {
              n147 = expression code="10**(x/20 )/2"(w371) -> (w369:sgl)
              n148 = expression code="2**(x-1)"(w370) -> (w368:i16)
              n149 = Divide(x=w369, y=w368) -> (x/y=w364:sgl)
              n150 = Multiply(x=w364, y=w367) -> (x*y=w366:dbl[][])
            }
            frame 2 {
              n151 = Negate(x=w380) -> (-x=w381:sgl)
              n152 = expression code="2**(x-1)"(w378) -> (w376:i16)
              n153 = Compound Arithmetic op=ADD(w383, w381, w382) -> (w379:sgl)
              n154 = expression code="10**(x/20 )/2"(w379) -> (w377:sgl)
              n155 = Divide(x=w377, y=w376) -> (x/y=w375:sgl)
              n156 = Multiply(x=w375, y=w374) -> (x*y=w373:dbl[][])
            }
            frame 3 {
              n157 = expression code="10**(x/20 )/2"(w385) -> (w390:dbl)
              n158 = expression code="2**(x-1)"(w391) -> (w389:i16)
              n159 = Divide(x=w390, y=w389) -> (x/y=w388:dbl)
              n160 = Multiply(x=w388, y=w387) -> (x*y=w386:dbl[][])
            }
          }
          n161 = Subtract(x=w253, y=w289) -> (x-y=w340:dbl)
          n162 = Subtract(x=w310, y=w289) -> (x-y=w313:dbl)
          n163 = Subtract(x=w309, y=w289) -> (x-y=w312:dbl)
          n164 = Subtract(x=w253, y=w255) -> (x-y=w254:dbl)
          n165 = Subtract(x=w255, y=w289) -> (x-y=w341:dbl)
          n166 = Divide(x=w341, y=w288) -> (x/y=w334:dbl)
          n167 = expression code="x/2"(w254) -> (w258:dbl)
          n168 = Divide(x=w257, y=w287) -> (x/y=w342:dbl)
          n169 = Divide(x=w340, y=w288) -> (x/y=w339:dbl)
          n170 = Divide(x=w313, y=w288) -> (x/y=w304:dbl)
          n171 = Divide(x=w259, y=w287) -> (x/y=w326:dbl)
          n172 = Divide(x=w306, y=w287) -> (x/y=w314:dbl)
          n173 = Divide(x=w312, y=w288) -> (x/y=w311:dbl)
          n174 = Add(x=w253, y=w258) -> (x+y=w256:dbl)
          n175 = Divide(x=w305, y=w287) -> (x/y=w303:dbl)
          n176 = Subtract(x=w339, y=w334) -> (x-y=w324:dbl)
          n177 = Subtract(x=w311, y=w304) -> (x-y=w302:dbl)
          n178 = Subtract(x=w342, y=w326) -> (x-y=w323:dbl)
          n179 = Subtract(x=w314, y=w303) -> (x-y=w301:dbl)
          n180 = Array Subset(array=w264, index (row)=w334, length (row)=w324, index (col)=w326, length (col)=w323) -> (w283:dbl[][])
          n181 = Array Subset(array=w263, index (row)=w304, length (row)=w302, index (col)=w303, length (col)=w301) -> (w284:dbl[][])
          n182 = Strip Path(path=w317) -> (stripped path=w319:path, name=w322:string)
          n183 = for {
            tunnel: w298 -> [w354]
            tunnel: w283 -> [w353] mode=indexing
            tunnel: [w352] -> w280 mode=indexing
            # "Envelope"
            n184 = call <vilib>:"Fast Hilbert Transform.vi"("X"=w353) -> ("Hilbert{X}"=w356:dbl[])  [unwired: 1 out]
            n185 = Re/Im To Complex(1:w356, 2:w353) -> (0:w355:cdb[])
            n186 = Absolute Value(x=w355) -> (abs(x)=w351:dbl[])
            n187 = Multiply(x=w354, y=w351) -> (x*y=w352:dbl[])
          }
          n188 = for {
            tunnel: w298 -> [w348]
            tunnel: w284 -> [w347] mode=indexing
            tunnel: [w346] -> w276 mode=indexing
            n189 = call <vilib>:"Fast Hilbert Transform.vi"("X"=w347) -> ("Hilbert{X}"=w350:dbl[])  [unwired: 1 out]
            n190 = Re/Im To Complex(1:w350, 2:w347) -> (0:w349:cdb[])
            n191 = Absolute Value(x=w349) -> (abs(x)=w345:dbl[])
            n192 = Multiply(x=w348, y=w345) -> (x*y=w346:dbl[])
          }
          n193 = Build Path(base path=w319, name or relative path="RMSValuesInFlowA.txt" ("file path (dialog if empty)")) -> (appended path=w316:path)
          n194 = Array Size(array=w280) -> (size(s)=w282:i32[])
          n195 = Array Size(array=w283) -> (size(s)=w344:i32[])
          n196 = Array Size(array=w276) -> (size(s)=w278:i32[])
          n197 = Array Size(array=w284) -> (size(s)=w300:i32[])
          n198 = Multiply Array Elements(1:w282) -> (0:w281:i32)
          n199 = Multiply Array Elements(1:w344) -> (0:w343:i32)
          n200 = Multiply Array Elements(1:w278) -> (0:w277:i32)
          n201 = Multiply Array Elements(1:w300) -> (0:w299:i32)
          n202 = Reshape Array(w280, w281) -> (w279:dbl[])
          n203 = Reshape Array(w283, w343) -> (w272:dbl[])
          n204 = Reshape Array(w276, w277) -> (w275:dbl[])
          n205 = Reshape Array(w284, w299) -> (w273:dbl[])
          n206 = call-poly <vilib>:"RMS.vi"("X"=w272) -> ("rms value"=w325:dbl)  [unwired: 1 out]
          n207 = call <vilib>:"Std Deviation and Variance.vi"("X"=w279) -> ("mean"=w269:dbl, "variance"=w268:dbl)  [unwired: 1 in, 1 out]
          n208 = call-poly <vilib>:"RMS.vi"("X"=w273) -> ("rms value"=w297:dbl)  [unwired: 1 out]
          n209 = call <vilib>:"Std Deviation and Variance.vi"("X"=w275) -> ("mean"=w267:dbl, "variance"=w266:dbl)  [unwired: 1 in, 1 out]
          n210 = expression code="20*log(x)"(w325) -> (w285:dbl)
          "RMS flow dB" <- w285
          n211 = Array Size(array=w273) -> (size(s)=w271:i32)
          "Pts BG" <- w271
          n212 = Subtract(x=w267, y=w269) -> (x-y=w293:dbl)
          n213 = expression code="20*log(x)"(w297) -> (w291:dbl)
          "RMS dB BG" <- w291
          n214 = Add(x=w268, y=w266) -> (x+y=w295:dbl)
          n215 = local read "ROI (mm)"() -> (w262:T9)
          n216 = Square Root(x=w295) -> (sqrt(x)=w294:dbl)
          n217 = Subtract(x=w285, y=w291) -> (x-y=w286:dbl)
          "dB CBR" <- w286
          n218 = Divide(x=w293, y=w294) -> (x/y=w290:dbl)
          "CNR" <- w290
          n219 = Bundle("mean"=w269, "variance"=w268, "mean"=w267, "variance"=w266) -> (→"Values":T8)  [unwired: 1 in]
          n220 = Array Size(array=w272) -> (size(s)=w270:i32)
          "Pts  flow" <- w270
          n221 = Unbundle By Name(w262) -> ("X"=w261:dbl, "Y"=w260:dbl)
          n222 = Build Array(w285, w291, w286, w290, w269, w268, w267, w266, w270, w271, w261, w260, w256) -> (w296:dbl[])
          n223 = Number To Fractional String(number=w296) -> (F-format string=w321:string[])  [unwired: 3 in]
          n224 = Build Array (concatenate)(w322, w321) -> (w320:string[])
          n225 = case shown="True" "Save RMS" {
            tunnel: w320 -> [_ w361]
            tunnel: w316 -> [_ w360]
            tunnel: [_ w358] -> _
            frame False {
            }
            frame True {
              n226 = call-poly <vilib>:"Write Delimited Spreadsheet.vi"("file path (dialog if empty)"=w360, "1D data"=w361, "append to file? (new file:F)"=TRUE) -> ("error out"=w358:errorcluster)  [unwired: 11 in, 1 out]
            }
          }
        }
        event "Save RF in window", "row to show": Value Change {
          # "Take window"
          # "Scale accordingly"
          n227 = event-data() -> ()  [unwired: 7 out]
          n228 = Unbundle By Name(w417) -> ("RF Info.RF file att"=w438:string)
          n229 = Unbundle By Name(w417) -> ("Votage scaling.Digitizer (dB)"=w423:sgl, "Votage scaling.Gain (dB)"=w427:sgl, "Votage scaling.Atten (dB)"=w425:sgl)
          n230 = local read "Vert Scale"() -> (w397:u16)
          n231 = Unbundle By Name(w417) -> ("A/D info.# A/D bits"=w426:i16)
          n232 = Fract/Exp String To Number(string=w438) -> (number=w418:dbl)  [unwired: 4 out]
          n233 = Unbundle By Name(w417) -> ("A/D info.sample rate MHz"=w411:u16, "Votage scaling.Digitizer (dB)"=w419:sgl, "Votage scaling.Gain (dB)"=w420:sgl, "Votage scaling.Atten (dB)"=w421:sgl)  [unwired: 1 out]
          n234 = Transpose 2D Array(2D array=w396) -> (transposed array=w424:dbl[][])
          n235 = property on="Raw data" class="IntGraph (strict)"() -> ("XScale.Offset"=w437:dbl, "XScale.Multiplier"=w436:dbl, "YScale.Multiplier"=w435:dbl)  [unwired: 2 in, 2 out]
          n236 = property on="Raw data" class="IntGraph (strict)"("Active Cursor"=u32 0 ("Write Attribute"), "Active Cursor"=u32 1 ("Write Attribute")) -> ("Cursor.Cursor X"=w434:dbl, "Cursor.Cursor Y"=w430:dbl, "Cursor.Cursor X"=w433:dbl, "Cursor.Cursor Y"=w429:dbl)  [unwired: 2 in, 2 out]
          n237 = case shown="0, Default" w397 {
            tunnel: w426 -> [_ w467 w474 w486]
            tunnel: w423 -> [_ w468 w479 _]
            tunnel: w425 -> [_ _ w478 _]
            tunnel: w427 -> [_ _ w476 _]
            tunnel: w424 -> [w461 w463 w470 w482]
            tunnel: [w461 w462 w469 w481] -> w416
            tunnel: w418 -> [_ _ _ w480]
            frame 0, Default {
              (unwired) 1
            }
            frame 1 {
              (unwired) 1000
              n238 = expression code="10**(x/20 )/2"(w468) -> (w466:sgl)
              n239 = expression code="2**(x-1)"(w467) -> (w465:i16)
              n240 = Divide(x=w466, y=w465) -> (x/y=w464:sgl)
              n241 = Multiply(x=w464, y=w463) -> (x*y=w462:dbl[][])
            }
            frame 2 {
              (unwired) 1000
              n242 = Negate(x=w476) -> (-x=w477:sgl)
              n243 = expression code="2**(x-1)"(w474) -> (w472:i16)
              n244 = Compound Arithmetic op=ADD(w479, w477, w478) -> (w475:sgl)
              n245 = expression code="10**(x/20 )/2"(w475) -> (w473:sgl)
              n246 = Divide(x=w473, y=w472) -> (x/y=w471:sgl)
              n247 = Multiply(x=w471, y=w470) -> (x*y=w469:dbl[][])
            }
            frame 3 {
              (unwired) 1000
              n248 = expression code="10**(x/20 )/2"(w480) -> (w485:dbl)
              n249 = expression code="2**(x-1)"(w486) -> (w484:i16)
              n250 = Divide(x=w485, y=w484) -> (x/y=w483:dbl)
              n251 = Multiply(x=w483, y=w482) -> (x*y=w481:dbl[][])
            }
          }
          n252 = Negate(x=w420) -> (-x=w422:sgl)
          n253 = Subtract(x=w433, y=w437) -> (x-y=w440:dbl)
          n254 = Subtract(x=w434, y=w437) -> (x-y=w441:dbl)
          n255 = Compound Arithmetic op=ADD(w419, w422, w421) -> ()  [unwired: 1 out]
          n256 = Divide(x=w441, y=w436) -> (x/y=w428:dbl)
          n257 = Divide(x=w430, y=w435) -> (x/y=w442:dbl)
          n258 = Divide(x=w440, y=w436) -> (x/y=w439:dbl)
          n259 = Divide(x=w429, y=w435) -> (x/y=w415:dbl)
          n260 = Reciprocal(x=w411) -> (1/x=w412:dbl)
          n261 = Subtract(x=w439, y=w428) -> (x-y=w413:dbl)
          n262 = Subtract(x=w442, y=w415) -> (x-y=w410:dbl)
          n263 = expression code="x/2"(w410) -> (w408:dbl)
          n264 = Array Subset(array=w416, index (row)=w428, length (row)=w413, index (col)=w415, length (col)=w410) -> (w414:dbl[][])
          n265 = Transpose 2D Array(2D array=w414) -> (transposed array=w398:dbl[][])
          n266 = for {
            N: w413 -> [_]
            tunnel: w412 -> [w460]
            tunnel: [w458] -> w406 mode=indexing
            i -> [w459]
            n267 = Multiply(x=w459, y=w460) -> (x*y=w458:dbl)
          }
          n268 = for {
            N: w408 -> [_]
            tunnel: w398 -> [w455]
            tunnel: [w454] -> w407 mode=indexing
            i -> [w457]
            n269 = Multiply(x=2, y=w457) -> (x*y=w452:i32)
            n270 = Increment(x=w452) -> (x+1=w453:i32)
            n271 = Index Array(array=w455, index (row)=w452) -> (element=w447:dbl[])  [unwired: 1 in]
            n272 = Index Array(array=w455, index (row)=w453) -> (element=w446:dbl[])  [unwired: 1 in]
            n273 = call <vilib>:"Fast Hilbert Transform.vi"("X"=w446) -> ("Hilbert{X}"=w451:dbl[])  [unwired: 1 out]
            n274 = call <vilib>:"Fast Hilbert Transform.vi"("X"=w447) -> ("Hilbert{X}"=w449:dbl[])  [unwired: 1 out]
            n275 = Re/Im To Complex(1:w451, 2:w446) -> (0:w450:cdb[])
            n276 = Re/Im To Complex(1:w449, 2:w447) -> (0:w448:cdb[])
            n277 = Absolute Value(x=w450) -> ()  [unwired: 1 out]
            n278 = Absolute Value(x=w448) -> ()  [unwired: 1 out]
            n279 = Add(x=w447, y=w446) -> (x+y=w454:dbl[])
          }
          n280 = Strip Path(path=w409) -> (stripped path=w401:path, name=w405:string)
          n281 = Search and Replace String(input string=w405, search string=".eye", replace string=".txt" ("replace string (\"\")")) -> (result string=w402:string)  [unwired: 5 in, 3 out]
          n282 = Build Path(base path=w401, name or relative path=w402) -> (appended path=w400:path)
          n283 = Build Array (concatenate)(w406, w398, w407) -> (w395:dbl[][])
          n284 = Index Array(array=w395, index (row)="row to show") -> (element=→"Waveform Graph 3":dbl[])  [unwired: 1 in]
          n285 = case shown="True" TRUE {
            tunnel: w395 -> [_ w445]
            tunnel: w400 -> [_ w443]
            frame False {
            }
            frame True {
              n286 = call-poly <vilib>:"Write Delimited Spreadsheet.vi"("file path (dialog if empty)"=w443, "2D data"=w445, "transpose? (no:F)"=TRUE) -> ()  [unwired: 11 in, 2 out]
            }
          }
        }
        event "View Header?": Value Change {
          n287 = event-data() -> ()  [unwired: 2 out]
          n288 = call "ReadHeadFast.vi"("new file path"=w489) -> ("refnum out"=w488:refnum<file>)  [unwired: 7 in, 3 out]
          n289 = Close File(refnum=w488) -> ()  [unwired: 1 in, 2 out]
        }
        event Value Change {
          n290 = event-data() -> ("NewVal"=w505:T10)  [unwired: 1 out]
          n291 = Unbundle By Name(w493) -> ("Scan Info"=w495:T1, "ROI Box"=w499:u16[], "Patient Info.previously\nscanned"=w498:string)
          n292 = Unbundle By Name(w493) -> ("A/D info.# A/D bits"=w502:i16)
          n293 = Equal?(x=w498, y="F") -> (x = y?=w497:bool)
          n294 = case shown="True" w497 {
            tunnel: w503 -> [_ w513]
            tunnel: w499 -> [_ w512]
            tunnel: w491 -> [_ w510]
            tunnel: w495 -> [_ w509]
            tunnel: w494 -> [_ w508]
            frame False {
            }
            frame True {
              # "Add in for flotare cals"
              n295 = call "FloaterCalc.vi"("Log"=w508, "medians"="medians", "left rank"="left rank", "ROI Box"=w512, "Scan Info"=w509, "new path in"=w513, "Raw Data In"=w510) -> ("Masked Data"=→"Raw data 2":dbl[][], "RMS noise x6"=w511:dbl)  [unwired: 11 in]
              n296 = property on="Raw data 2" class="IntGraph (strict)"("ZScale.Maximum"=w511) -> ()  [unwired: 2 in, 2 out]
              n297 = property on="dB 2" class="IntGraph (strict)"("ZScale.Maximum"=w511) -> ()  [unwired: 2 in, 2 out]
            }
          }
          n298 = To Double Precision Float(number=w502) -> (double precision float=w501:dbl)
          n299 = expression code="20*log(2**(x-1))"(w501) -> (w500:dbl)
          n300 = case shown="\"Linear Color Scale\"" w505 {
            tunnel: [w520 w524 w525 w528 w531] -> w504
            tunnel: w491 -> [w521 w523 w525 w529 w532]
            tunnel: w502 -> [_ w522 _ _ w530]
            tunnel: w493 -> [_ _ _ w527 _]
            frame "Linear Abs Grey", Default {
              n301 = Absolute Value(x=w521) -> (abs(x)=w520:dbl[][])
            }
            frame "Log Grey Scale" {
              n302 = call "LogScaleImage.vi"("A/D bits"=w522, "input array"=w523) -> ("log scale image"=w524:dbl[][])  [unwired: 1 out]
            }
            frame "Linear Color Scale" {
            }
            frame "Verasonics Doppler" {
              n303 = call "DopplerScale.vi"("Header In"=w527, "Velocity index in"=w529) -> ("max doppler velocity cm/s"=→"max doppler velocity mm/s":dbl, "Velocity Out"=w528:dbl[][])  [unwired: 6 in, 2 out]
            }
            frame "dB Scale" {
              n304 = call "dBScale.vi"("Bit Depth"=w530, "Data In"=w532) -> ("Data Out"=w531:dbl[][])  [unwired: 3 in]
            }
          }
          n305 = case shown="True" "Scale" {
            tunnel: w502 -> [_ w518]
            tunnel: w505 -> [_ w517]
            frame False {
            }
            frame True {
              n306 = call "SetScale.vi"("# A/D bits"=w518, "Display mode"=w517) -> ("Array"=w519:cluster{dbl, u32}[])
              n307 = property on="Raw data" class="IntGraph (strict)"("ZScale.MarkerVals[]"=w519) -> ()  [unwired: 2 in, 2 out]
            }
          }
          n308 = call "HilbertLogCompress.vi"("Array in"=w491) -> ()  [unwired: 10 in, 1 out]
          n309 = expression code="20*log(abs(x))"(w491) -> (w490:dbl[][])
          "dB" <- w490
          "dB 2" <- w490
          n310 = Array Max & Min(array=w490) -> ()  [unwired: 4 out]
          n311 = Subtract(x=w490, y=w500) -> ()  [unwired: 1 out]
          n312 = Transpose 2D Array(2D array=w504) -> (transposed array=→"Raw data":dbl[][])
        }
        event "Slide": Value Change {
          # "Will auto adjst range dB scale figure."
          n313 = event-data() -> ()  [unwired: 7 out]
          n314 = Unbundle("Slide") -> (w535:dbl, w534:dbl)
          n315 = property on="dB" class="IntGraph (strict)"("ZScale.Maximum"=w535, "ZScale.Minimum"=w534) -> ()  [unwired: 2 in, 2 out]
        }
        event "Axis scaling", "One Way": Value Change {
          (unwired) T19 {"Offset"=0.0, "Multiplier"=0.0} ("X Scale.Offset and Multiplier")
          n316 = event-data() -> ()  [unwired: 2 out]
          n317 = call "Get_Plot_Scales.vi"("Header In"=w541, "Sound Speed modify"=w542, "One Way"="One Way", "Axis scaling"="Axis scaling") -> ("Depth Scale"=w539:cluster{"start depth":dbl, "depth interval":dbl}, "Width Scale"=w538:cluster{"Start":dbl, "width Interval":dbl})  [unwired: 10 in]
          n318 = property on="Blow up of blue Line" class="WFGraph (strict)"("XScale.Ofst&Mult"=w539) -> ()  [unwired: 2 in, 2 out]
          n319 = property on="dB" class="IntGraph (strict)"("XScale.Ofst&Mult"=w538, "YScale.Ofst&Mult"=w539) -> ()  [unwired: 2 in, 2 out]
          n320 = property on="Raw data" class="IntGraph (strict)"("XScale.Ofst&Mult"=w539, "YScale.Ofst&Mult"=w538) -> ()  [unwired: 2 in, 2 out]
          n321 = property on="Match Data" class="IntGraph (strict)" props=["XScale", "Ofst&Mult", "YScale", "Ofst&Mult", "XScale", "Ofst&Mult"]("XScale.Ofst&Mult"=w538, "YScale.Ofst&Mult"=w539) -> ()  [unwired: 2 in, 3 out]
        }
        event "Save BMP?": Value Change {
          w546 = -55.0 ("ZScale.Minimum")
          # "Create BMP file"
          n322 = event-data() -> ()  [unwired: 7 out]
          n323 = property on="Sector as data array" class="IntGraph (strict)" props=["Color Table", "Z Scale", "Range:Maximum", "Z Scale", "Range:Minimum"]() -> ("Color Table"=w552:u32[], "Z Scale.Range:Maximum"=w547:dbl)  [unwired: 2 in, 3 out]
          n324 = local read "Sector as data array"() -> (w548:dbl[][])
          n325 = for {
            tunnel: w547 -> [w567]
            tunnel: w546 -> [w566]
            tunnel: w548 -> [w565] mode=indexing
            tunnel: [w564] -> w559 mode=indexing
            n326 = call <vilib>:"Y[i]=Clip{X[i]}.vi"("lower limit"=w566, "upper limit"=w567, "Input Array"=w565) -> ("Clipped Array"=w564:dbl[])  [unwired: 1 out]
          }
          n327 = Subtract(x=w559, y=w546) -> (x-y=w558:dbl[][])
          n328 = call <vilib>:"Quick Scale 2D.vi"("X"=w558) -> ("Yij=Xij/Max|X|"=w557:dbl[][])  [unwired: 2 out]
          n329 = Multiply(x=255, y=w557) -> (x*y=w555:dbl[][])
          n330 = for {
            tunnel: w555 -> [w563] mode=indexing
            tunnel: [w562] -> w556 mode=indexing
            n331 = Reverse 1D Array(array=w563) -> (reversed array=w562:dbl[])
          }
          n332 = local read "cursor"() -> (w551:dbl)
          n333 = Transpose 2D Array(2D array=w556) -> (transposed array=w545:dbl[][])
          n334 = local read "Pixels in x"() -> (w550:i16)
          n335 = Add(x=w551, y=w551) -> (x+y=w554:dbl)
          n336 = Subtract(x=w550, y=w554) -> (x-y=w553:dbl)
          n337 = Array Subset(array=w545, index (col)=w551, length (col)=w553) -> ()  [unwired: 2 in, 1 out]
          n338 = call <vilib>:"Flatten Pixmap.vi"("colors"=w552, "8-bit pixmap"=w545) -> ("image data"=w560:T20)  [unwired: 4 in, 5 out]
          n339 = File Dialog() -> (3:w561:path)  [unwired: 1 in, 9 out]
          n340 = call <vilib>:"Write BMP File.vi"("image data"=w560, "path to BMP file"=w561) -> ()  [unwired: 1 in, 9 out]
        }
        event "Create Sector", "Pixels in x", "Pixels in y", "Add Lines", "Reduce x data factor", "Smooth factor": Value Change {
          w580 = u8 1 ("X Scale.Scale Fit")
          # "Set up scaling for sector image"
          # "If Prostate or Rectal exam,\nconvert to sector image also."
          # "perform sector conversion"
          n341 = event-data() -> ()  [unwired: 2 out]
          n342 = Unbundle By Name(w608) -> ("A/D info.# A/D bits"=w572:i16, "Scan Info.sector scan angle"=w600:sgl, "A/D info.sample rate MHz"=w601:u16, "Scan Info"=w607:T1)
          "Scan Info" <- w607
          n343 = Equal?(x=w600, y=360) -> (x = y?=w620:bool)
          n344 = Select(t="Pixels in x", s=w620, f="Pixels in y") -> (s? t:f=w622:i16)
          n345 = Reciprocal(x=w601) -> (1/x=w619:dbl)
          n346 = property on="Sector as data array" class="IntGraph (strict)"() -> ("Plot Bounds"=w577:T11, "Plot Area Size"=w578:T12)  [unwired: 2 in, 2 out]
          n347 = call "ConvertToSec.vi"("raw image data in"=w595, "reduce pts by factor of"="Reduce x data factor", "Add Lines"="Add Lines", "pixels in x"="Pixels in x", "pixels in y"=w622, "Time between rf pts\nmicros"=w619, "Scan Info"=w607, "Smooth factor"="Smooth factor", "use min z value?"=FALSE) -> ("raw sector out"=w598:dbl[][], "Axis scaling Params"=w609:T6, "scales"=w605:cluster{"inc x (mm)":dbl, "inc y (mm)":dbl})  [unwired: 3 in, 5 out]
          "Axis scaling Params" <- w609
          n348 = Unbundle(T12 {"Width"=350, "Height"=333} ("Plot Area:Size")) -> ("Width"=w592:u32, "Height"=w594:u32)
          n349 = expression code="20*log(x)"(w598) -> (w597:dbl[][])
          n350 = Unbundle By Name(w605) -> ("inc x (mm)"=w583:dbl, "inc y (mm)"=w582:dbl)
          "inc y (mm)" <- w582
          "inc x (mm)" <- w583
          n351 = Multiply(x="Pixels in x", y=w583) -> (x*y=w586:dbl)
          n352 = Multiply(x=w582, y="Pixels in y") -> (x*y=w587:dbl)
          n353 = Divide(x=w592, y=w586) -> (x/y=w588:dbl)
          n354 = Divide(x=w594, y=w587) -> (x/y=w589:dbl)
          n355 = Unbundle By Name(w609) -> ("X right"=w618:dbl, "X left"=w617:dbl, "Y high"=w570:dbl)
          n356 = property on="Sector as data array" class="IntGraph (strict)"() -> ("Cursor.Cursor Position:Cursor X"=w611:dbl)  [unwired: 2 in, 2 out]
          n357 = Divide(x=w588, y=w589) -> (x/y=w593:dbl)
          n358 = Subtract(x=w618, y=w617) -> (x-y=w616:dbl)
          n359 = Decrement(x=w572) -> (x-1=w574:i16)
          n360 = Array Max & Min(array=w597) -> ()  [unwired: 4 out]
          n361 = Greater?(x=w593, y=1.0) -> (0:w590:bool)
          n362 = Absolute Value(x=w570) -> (abs(x)=w569:dbl)
          n363 = Divide(x=w611, y=w616) -> (x/y=w615:dbl)
          n364 = Power Of 2(x=w574) -> (2^x=w573:dbl)
          n365 = case shown="False" w590 {
            tunnel: w592 -> [_ w636]
            tunnel: w593 -> [w629 w635]
            tunnel: w594 -> [w628 _]
            tunnel: T11 {"Left"=499, "Top"=34, "Right"=884, "Bottom"=389} ("Plot Area Bounds") -> [w623 w634]
            tunnel: [w624 w630] -> w581
            tunnel: w577 -> [_ _]
            tunnel: w578 -> [_ _]
            frame False {
              n366 = Unbundle By Name(w623) -> ("Top"=w627:i16)
              n367 = Multiply(x=w628, y=w629) -> (x*y=w625:dbl)
              n368 = Add(x=w627, y=w625) -> (x+y=w626:dbl)
              n369 = Bundle By Name(cluster=w623, "Bottom"=w626) -> (w624:T11)
            }
            frame True {
              n370 = Unbundle By Name(w634) -> ("Left"=w632:i16)
              n371 = Divide(x=w636, y=w635) -> (x/y=w633:dbl)
              n372 = Add(x=w632, y=w633) -> (x+y=w631:dbl)
              n373 = Bundle By Name(cluster=w634, "Right"=w631) -> (w630:T11)
            }
          }
          n374 = Multiply(x=w615, y="Pixels in x") -> (x*y=w612:dbl)
          n375 = case shown="True" TRUE {
            tunnel: w583 -> [_ w642]
            tunnel: [w639 w642] -> w614
            tunnel: [w639 w641] -> w613
            tunnel: w582 -> [_ w641]
            tunnel: w612 -> [_ w640]
            tunnel: [w638 w640] -> w610
            tunnel: w611 -> [w638 _]
            tunnel: [FALSE ("Create Sector") _] -> w596
            frame False {
              w639 = 1
            }
            frame True {
            }
          }
          "cursor" <- w610
          n376 = expression code="20*log(x)"(w573) -> (w571:dbl)
          n377 = Subtract(x=w597, y=w571) -> (x-y=→"Sector as data array":dbl[][])
          n378 = local write "Create Sector"(w596) -> ()
          n379 = property on="Sector as data array" class="IntGraph (strict)"("X Scale.Offset and Multiplier:Multiplier"=w614, "Y Scale.Offset and Multiplier:Multiplier"=w613, "YScale.Offset"=w569) -> ()  [unwired: 2 in, 2 out]
          n380 = property on="Sector as data array" class="IntGraph (strict)" props=["XScale", "ScaleFit", "YScale", "ScaleFit", "Plot Bounds", "Plot Area Size"]("XScale.ScaleFit"=w580, "YScale.ScaleFit"=w580, "Plot Bounds"=w581) -> ()  [unwired: 2 in, 3 out]
        }
        event "new file path", "File Ext": Value Change {
          n381 = event-data() -> ()  [unwired: 7 out]
        }
        event "Save Spectra?": Value Change {
          (unwired) "test.txt" ("string")
          w649 = TRUE  # transpose
          w670 = FALSE  # append
          # "Save data referenced to 1 Vpp."
          # "Save Spectra to file"
          n382 = event-data() -> ()  [unwired: 3 out]
          n383 = Unbundle By Name(w659) -> ("A/D info.sample rate MHz"=w657:u16, "RF Info.RF file att"=w665:string)
          n384 = Strip Path(path=w669) -> (stripped path=w651:path, name=w656:string)
          n385 = Fract/Exp String To Number(string=w665) -> (number=w661:dbl)  [unwired: 4 out]
          n386 = local read "Spectrum"() -> (w674:T4)
          n387 = Reciprocal(x=w657) -> (1/x=w668:dbl)
          n388 = expression code="1000*pow(10,x/20)/256"(w661) -> (w664:dbl)
          n389 = Index Array(array=w674) -> (element=w673:T18)  [unwired: 1 in]
          n390 = local read "blue win"() -> (w663:dbl[])
          n391 = Unbundle(w673) -> ("df (MHz)"=w672:dbl, "Best Linear Fit"=w660:dbl[])  [unwired: 1 out]
          n392 = for {
            tunnel: w660 -> [_] mode=indexing
            tunnel: w672 -> [w684]
            tunnel: [w683] -> w671 mode=indexing
            i -> [w685]
            n393 = Multiply(x=w684, y=w685) -> (x*y=w683:dbl)
          }
          n394 = for {
            tunnel: w668 -> [w681]
            tunnel: [w680] -> w667 mode=indexing
            tunnel: w663 -> [_] mode=indexing
            i -> [w682]
            n395 = Multiply(x=w681, y=w682) -> (x*y=w680:dbl)
          }
          n396 = Search and Replace String(input string=w656, search string=".eye", replace string=".txt" ("replace string (\"\")")) -> (result string=w646:string)  [unwired: 5 in, 3 out]
          n397 = Multiply(x=w663, y=w664) -> (x*y=w662:dbl[])
          n398 = case shown="False" "Drop freq coumn?" {
            tunnel: w671 -> [w677 _]
            tunnel: w660 -> [w676 w679]
            tunnel: [w675 w678] -> w658
            frame False {
              n399 = Build Array(w677, w676) -> (w675:dbl[][])
            }
            frame True {
              n400 = Build Array(w679) -> (w678:dbl[][])
            }
          }
          n401 = Concatenate Strings("AllAvg" ("string"), "Spec" ("string"), w646) -> (w652:string)
          n402 = Build Array(w667, w662) -> (w666:dbl[][])
          n403 = Build Array (concatenate)(w666, w658) -> ()  [unwired: 1 out]
          n404 = Build Path(base path=w651, name or relative path=w652) -> (appended path=w650:path)
          n405 = call-poly <vilib>:"Write Delimited Spreadsheet.vi"("file path (dialog if empty)"=w650, "2D data"=w658, "append to file? (new file:F)"=w670, "transpose? (no:F)"=w649) -> ()  [unwired: 10 in, 2 out]
        }
        event "Save RF": Value Change {
          # "Save Spectra to file"
          n406 = event-data() -> ()  [unwired: 2 out]
          n407 = Unbundle By Name(w699) -> ("A/D info.sample rate MHz"=w698:u16)
          n408 = Strip Path(path=w692) -> (stripped path=w694:path, name=w691:string)
          n409 = local read "Blow up of blue Line"() -> (w705:dbl[][])
          n410 = Reciprocal(x=w698) -> (1/x=w704:dbl)
          n411 = Index Array(array=w705) -> (element=w702:dbl[])  [unwired: 2 in]
          n412 = for {
            tunnel: w702 -> [_] mode=indexing
            tunnel: w704 -> [w707]
            tunnel: [w706] -> w703 mode=indexing
            i -> [w708]
            n413 = Multiply(x=w707, y=w708) -> (x*y=w706:dbl)
          }
          n414 = Search and Replace String(input string=w691, search string=".eye", replace string=".txt" ("replace string (\"\")")) -> (result string=w688:string)  [unwired: 5 in, 3 out]
          n415 = Build Array(w703, w702) -> (w700:dbl[][])
          n416 = Concatenate Strings("RF" ("string"), w688) -> (w690:string)
          n417 = Concatenate Strings("RF" ("string"), "test.txt" ("string")) -> ()  [unwired: 1 out]
          n418 = Build Path(base path=w694, name or relative path=w690) -> (appended path=w689:path)
          n419 = call-poly <vilib>:"Write Delimited Spreadsheet.vi"("file path (dialog if empty)"=w689, "2D data"=w700, "transpose? (no:F)"=TRUE) -> ()  [unwired: 11 in, 2 out]
        }
        event "Next File in Dir?", "Delete File": Value Change {
          # "Increment by one file in directory"
          n420 = event-data() -> ()  [unwired: 7 out]
          n421 = property on="new file path" class="Path"() -> ("MatchPttn"=w716:string)  [unwired: 2 in, 2 out]
          n422 = Strip Path(path=w713) -> (stripped path=w714:path, name=w724:string)
          n423 = local write "Next File in Dir?"(FALSE ("Next File in Dir?")) -> ()
          n424 = List Folder(path=w714, pattern=w716) -> (path out=w715:path, filenames=w718:string[])  [unwired: 1 in, 3 out]
          n425 = Search 1D Array(1D array=w718, element=w724) -> (index of element=w723:i32)  [unwired: 1 out]
          n426 = Increment(x=w723) -> (x+1=w722:i32)
          n427 = Index Array(array=w718, index=w722) -> (element=w721:string)
          n428 = Build Path(base path=w715, name or relative path=w721) -> (appended path=w711:path)
          n429 = case shown="True" "Delete File" {
            tunnel: w713 -> [_ w726]
            tunnel: w711 -> [_ _]
            frame False {
            }
            frame True {
              n430 = Delete(path (use dialog)=w726, confirm (F)=FALSE) -> ()  [unwired: 1 in, 5 out]
            }
          }
          n431 = call <vilib>:"Check if File or Folder Exists.vi"("path"=w711) -> ("file or folder exists?"=w719:bool, "dup path"=w720:path)  [unwired: 1 in, 8 out]
          n432 = case shown="False" w719 {
            tunnel: w720 -> [_ w732]
            tunnel: w718 -> [w731 _]
            tunnel: w715 -> [w730 _]
            tunnel: [w728 w732] -> w717
            frame False {
              # "Handle last to first case"
              n433 = Index Array(array=w731) -> (element=w729:string)  [unwired: 1 in]
              n434 = Build Path(base path=w730, name or relative path=w729) -> (appended path=w728:path)
            }
            frame True {
            }
          }
          n435 = local write "new file path"(w717) -> ()
        }
        event Key Down {
          n436 = event-data() -> ("VKey"=w734:T21, "Char"=w735:i16)  [unwired: 1 out]
          n437 = case shown="\"ASCII\", Default" w734 {
            tunnel: w735 -> [w736 _ _]
            frame "ASCII", Default {
              n438 = case shown="88, 120" w736 {
                frame Default {
                }
                frame 88, 120 {
                  n439 = property on="Raw data" class="IntGraph (strict)"("XScale.ScaleFit"=u8 1 ("X Scale.Scale Fit")) -> ()  [unwired: 2 in, 2 out]
                }
                frame 89, 121 {
                  n440 = property on="Raw data" class="IntGraph (strict)"("YScale.ScaleFit"=u8 1 ("X Scale.Scale Fit")) -> ()  [unwired: 2 in, 2 out]
                }
              }
            }
            frame "Left" {
              n441 = property on="Prev File" class="Bool (strict)"("Val(Sgnl)"=TRUE ("Value (Signaling)")) -> ()  [unwired: 2 in, 2 out]
            }
            frame "Right" {
              n442 = property on="Next File in Dir?" class="Bool (strict)"("Val(Sgnl)"=TRUE ("Value (Signaling)")) -> ()  [unwired: 2 in, 2 out]
            }
          }
        }
        event "Prev File": Value Change {
          n443 = event-data() -> ()  [unwired: 7 out]
          n444 = property on="Prev File" class="Bool (strict)"("Value"=FALSE ("Prev File")) -> ()  [unwired: 2 in, 2 out]
          n445 = property on="new file path" class="Path"() -> ("MatchPttn"=w743:string)  [unwired: 2 in, 2 out]
          n446 = Strip Path(path=w751) -> (stripped path=w756:path, name=w755:string)
          n447 = List Folder(path=w756, pattern=w743) -> (path out=w746:path, filenames=w745:string[])  [unwired: 1 in, 3 out]
          n448 = Search 1D Array(1D array=w745, element=w755) -> (index of element=w754:i32)  [unwired: 1 out]
          n449 = Decrement(x=w754) -> (x-1=w753:i32)
          n450 = Index Array(array=w745, index=w753) -> (element=w752:string)
          n451 = Build Path(base path=w746, name or relative path=w752) -> (appended path=w747:path)
          n452 = call <vilib>:"Check if File or Folder Exists.vi"("path"=w747) -> ("file or folder exists?"=w748:bool, "dup path"=w749:path)  [unwired: 1 in, 8 out]
          n453 = case shown="False" w748 {
            tunnel: w749 -> [_ w762]
            tunnel: w745 -> [w761 _]
            tunnel: w746 -> [w760 _]
            tunnel: [w758 w762] -> w744
            frame False {
              # "Handle first to last case"
              n454 = Reverse 1D Array(array=w761) -> (reversed array=w757:string[])
              n455 = Index Array(array=w757) -> (element=w759:string)  [unwired: 1 in]
              n456 = Build Path(base path=w760, name or relative path=w759) -> (appended path=w758:path)
            }
            frame True {
            }
          }
          n457 = local write "new file path"(w744) -> ()
        }
        event "Header format": Value Change {
          n458 = event-data() -> ()  [unwired: 7 out]
        }
        event "Alter Header": Value Change {
          (unwired) T22 {"Energy (microJ)"=0, "Damping (In Ohm)"=0, "HP Filt(KHz) "=0, "LP Filt (MHz)"=0, "Gain (db)"=0, "prf (kHz)"=0.0, "Distance between\nscan lines (um)"=0, "Distance between\nscan planes (um)"=0, "Scan line gap (um)"=0.0, "Scan plane gap (um)"=0.0} ("Scan Settings")
          (unwired) T23 {"Energy (uJ or V)"=0, "Damp (Ohm) or Fc"=0, "HP Filt (KHz)"=0, "LP Filt (MHz)"=0, "Gain (db)"=0, "prf (kHz)"=0.0, "Distance between\nscan lines (um)"=0, "Distance between\nscan planes (um)"=0, "Scan line gap (um)"=0.0, "Scan plane gap (um)"=0.0} ("Scan Settings")
          n459 = event-data() -> ()  [unwired: 2 out]
          n460 = Strip Path(path=w789) -> (stripped path=w788:path)  [unwired: 1 out]
          n461 = Unbundle(w786) -> ("header info"=w776:cluster{"Header":string, "Head length":i16}, "A/D info"=w775:T24, "Tranducer Info"=w774:T25, "Scan Info"=w773:T1, "Time/Date Info"=w772:cluster{"date":string, "time":string}, "RF Info"=w771:T26, "Patient Info"=w770:T27, "Tissue Type"=w777:T28, "Votage scaling"=w778:T29, "Comment"=w779:string, "Misc Info"=w780:T30, "Therapy Parameters"=w781:T31, "Scan Settings"=w782:T23, "Compression Parameters"=w783:T32, "Patient Info Xtra"=w784:T33)  [unwired: 1 out]
          n462 = Bundle(cluster=T13 {"header info"={"Header"="", "Head length"=0}, "A/D info"={"# rf points per line"=0, "# lines per scan"=0, "sample rate MHz"=0, "# A/D bits"=0, "# bytes per A/D"=0, "TGC Flag"=0, "A/D Type"=""}, "Tranducer Info"={"bandwidth"=6.0, "center freq"=23.0, "start freq"=0.0, "ID"=6}, "Scan Info"={"delay"=0.0, "pivot distance"=0.0, "sector scan angle"=0.0, "operator"="", "Scan Mode"="", "location"=""}, "Time/Date Info"={"date"="", "time"=""}, "RF Info"={"RF file name"="", "RF file att"="", "RF cal file name"="", "RF cal file att"=""}, "Patient Info"={"ID"="test", "extended ID"="", "age"=0, "sex"="", "previously\nscanned"="N", "PSA"=0.0, "LOS"=1, "Ethnicty 2"=1, "Race"=4}, "Tissue Type"={"organ"=0, "disease type"=0, "disease location"=0, "IQ_pts"=0, "RcvBuffer"=0, "RcvFrame"=0, "IQBuff"=0, "IQFrame"=0, "IQPage"=0}, "Votage scaling"={"Digitizer (dB)"=0.0, "Gain (dB)"=40.0, "Atten (dB)"=3.0}, "Comment"="", "Misc Items"={"avg num"=0, "c speed"=0, "DivideBy"=0, "XMIT CHS"=0, "RCV CHS"=0, "Tx angle"=0}, "Therapy Parameters"={"Theraputic Freq (MHz)"=0.0, "Time on (s)"=0.0, "Therapy amplitude (mV)"=0.0, "Lines Before"=0, "Lines After"=0}, "Scan Settings"={"Energy (microJ)"=0, "Damping (In Ohm)"=0, "HP Filt(KHz) "=0, "LP Filt (MHz)"=0, "Gain (db)"=0, "prf (kHz)"=0.0, "Distance between\nscan lines (mm)"=0, "Distance between\nscan planes (mm)"=0, "prf (kHz) 2"=0.0, "prf (kHz) 3"=0.0}, "Compression Parameters"={"F1 (MHz)"=0.0, "F2 (MHz)"=0.0, "% taper"=0.0, "duration"=0.0}, "Patient Info Xtra"={"First Name"="", "Last Name"="", "Notes"=""}, "Boolean1"={FALSE, FALSE, FALSE, FALSE, FALSE, FALSE, FALSE, FALSE, FALSE, FALSE, TRUE, TRUE, FALSE, TRUE, FALSE, FALSE, FALSE, FALSE, FALSE, FALSE, FALSE, FALSE}, "Boolean2"={FALSE, FALSE, FALSE, FALSE, FALSE, FALSE, FALSE, FALSE, FALSE, FALSE, FALSE, FALSE, FALSE, FALSE, FALSE, FALSE, FALSE, FALSE, FALSE, FALSE, FALSE, FALSE, FALSE, FALSE, TRUE, TRUE, FALSE, FALSE, FALSE, FALSE, FALSE, FALSE, FALSE, FALSE, FALSE}, "Boolean3"={FALSE, FALSE, FALSE, FALSE, FALSE, FALSE, FALSE, FALSE, FALSE, FALSE, FALSE, FALSE, FALSE, FALSE, FALSE, FALSE, FALSE, FALSE, FALSE, FALSE, FALSE, FALSE}} ("Header In"), "header info"=w776, "A/D info"=w775, "Tranducer Info"=w774, "Scan Info"=w773, "Time/Date Info"=w772, "RF Info"=w771, "Patient Info"=w770, "Tissue Type"=w777, "Votage scaling"=w778, "Comment"=w779, "Misc Items"=w780, "Therapy Parameters"=w781, "Scan Settings"=w782, "Compression Parameters"=w783, "Patient Info Xtra"=w784, "Boolean1"=T14 {FALSE, FALSE, FALSE, FALSE, FALSE, FALSE, FALSE, FALSE, FALSE, FALSE, FALSE, FALSE, FALSE, FALSE, FALSE, FALSE, FALSE, FALSE, FALSE, FALSE, FALSE, FALSE}, "Boolean2"=T15 {FALSE, FALSE, FALSE, FALSE, FALSE, FALSE, FALSE, FALSE, FALSE, FALSE, FALSE, FALSE, FALSE, FALSE, FALSE, FALSE, FALSE, FALSE, FALSE, FALSE, FALSE, FALSE, FALSE, FALSE, FALSE, FALSE, FALSE, FALSE, FALSE, FALSE, FALSE, FALSE, FALSE, FALSE, FALSE}, "Boolean3"=T14 {FALSE, FALSE, FALSE, FALSE, FALSE, FALSE, FALSE, FALSE, FALSE, FALSE, FALSE, FALSE, FALSE, FALSE, FALSE, FALSE, FALSE, FALSE, FALSE, FALSE, FALSE, FALSE}) -> (w785:T13)
          n463 = call "AlterHeader.vi"("Header In"=w785, "Choose Directory"=w788) -> ()  [unwired: 2 out]
        }
        event "1-to-1": Value Change {
          n464 = event-data() -> ()  [unwired: 7 out]
          n465 = stacked-sequence {
            tunnel: w793 -> [w796 _]
            tunnel: w792 -> [_ w803]
            tunnel: w791 -> [w794 w802]
            frame #0 {
              w797 = u8 1 ("Y Scale.Scale Fit")
              n466 = stacked-sequence {
                tunnel: [w800 _] -> w795
                frame #0 {
                  n467 = Wait (ms)(milliseconds to wait=u32 25) -> ()  [unwired: 1 out]
                  n468 = property on="Axis scaling" class="Bool (strict)"("Val(Sgnl)"=TRUE ("Value (Signaling)")) -> (error out=w800:errorcluster)  [unwired: 2 in, 1 out]
                }
                frame #1 {
                }
              }
              n469 = property on="Property Node" class="IntGraph (strict)"(reference=w794, error in=w795, "Plot Bounds"=w796, "YScale.ScaleFit"=w797, "XScale.ScaleFit"=w797) -> ()  [unwired: 2 out]
            }
            frame #1 {
              n470 = property on="Property Node" class="IntGraph (strict)"(reference=w802) -> (reference out=w801:refnum<vi>, "X Scale.Offset and Multiplier:Multiplier"=w819:dbl, "Y Scale.Offset and Multiplier:Multiplier"=w818:dbl, "Plot Bounds"=w807:T11, "Plot Area Size"=w806:T12)  [unwired: 1 in, 1 out]
              n471 = Unbundle By Name(w803) -> ("A/D info.# rf points per line"=w805:u16, "A/D info.# lines per scan"=w804:u16)
              n472 = Multiply(x=w805, y=w819) -> (x*y=w817:dbl)
              n473 = Multiply(x=w818, y=w804) -> (x*y=w816:dbl)
              n474 = Unbundle(w806) -> ("Width"=w811:u32, "Height"=w809:u32)
              n475 = Divide(x=w811, y=w817) -> (x/y=w815:dbl)
              n476 = Divide(x=w809, y=w816) -> (x/y=w814:dbl)
              n477 = Divide(x=w815, y=w814) -> (x/y=w810:dbl)
              n478 = Greater?(x=w810, y=1.0) -> (0:w813:bool)
              n479 = case shown="True" w813 {
                tunnel: w811 -> [_ w833]
                tunnel: w810 -> [w826 w832]
                tunnel: w809 -> [w825 _]
                tunnel: w807 -> [w820 w831]
                tunnel: [w821 w827] -> w808
                frame False {
                  n480 = Unbundle By Name(w820) -> ("Top"=w824:i16)
                  n481 = Multiply(x=w825, y=w826) -> (x*y=w822:dbl)
                  n482 = Add(x=w824, y=w822) -> (x+y=w823:dbl)
                  n483 = Bundle By Name(cluster=w820, "Bottom"=w823) -> (w821:T11)
                }
                frame True {
                  n484 = Unbundle By Name(w831) -> ("Left"=w829:i16)
                  n485 = Divide(x=w833, y=w832) -> (x/y=w830:dbl)
                  n486 = Add(x=w829, y=w830) -> (x+y=w828:dbl)
                  n487 = Bundle By Name(cluster=w831, "Right"=w828) -> (w827:T11)
                }
              }
              n488 = property on="Property Node" class="IntGraph (strict)"(reference=w801, "Plot Bounds"=w808) -> ()  [unwired: 1 in, 2 out]
            }
          }
        }
        event "Fill": Value Change {
          n489 = event-data() -> ()  [unwired: 7 out]
          n490 = property on="Raw data" class="IntGraph (strict)"("Plot Bounds"=w835) -> ()  [unwired: 2 in, 2 out]
        }
        event "Flip X": Value Change {
          n491 = event-data() -> ()  [unwired: 7 out]
          n492 = property on="Property Node" class="IntGraph (strict)"(reference=w837, "XScale.Flipped"="Flip X") -> ()  [unwired: 1 in, 2 out]
        }
        event "Flip Y": Value Change {
          n493 = event-data() -> ()  [unwired: 7 out]
          n494 = property on="Property Node" class="IntGraph (strict)"(reference=w840, "YScale.Flipped"="Flip Y") -> ()  [unwired: 1 in, 2 out]
        }
        event "View Pics": Value Change {
          n495 = event-data() -> ()  [unwired: 2 out]
          n496 = Strip Path(path=w844) -> (stripped path=w843:path)  [unwired: 1 out]
          n497 = call "ViewPicts.vi"("Choose Directory"=w843) -> ()  [unwired: 8 out]
        }
        event "Add Switch Noise?": Value Change {
          n498 = event-data() -> ()  [unwired: 7 out]
        }
        event "Eye to BMP": Value Change {
          n499 = event-data() -> ()  [unwired: 2 out]
          n500 = Strip Path(path=w849) -> (stripped path=w848:path)  [unwired: 1 out]
          n501 = call "MakeEyeBMP.vi"("Choose Directory"=w848) -> ()  [unwired: 15 out]
        }
        event "Syn Focus": Value Change {
          n502 = event-data() -> ()  [unwired: 3 out]
          n503 = Strip Path(path=w852) -> (stripped path=w851:path)  [unwired: 1 out]
          n504 = call "SynthApp.vi"("Choose Directory"=w851) -> ()  [unwired: 15 in]
        }
        event "Whole Image": Value Change {
          n505 = event-data() -> ()  [unwired: 3 out]
          n506 = Strip Path(path=w855) -> (stripped path=w854:path)  [unwired: 1 out]
          n507 = call "WholeImageROIFit.vi"("Select directory with EYE files"=w854) -> ()  [unwired: 3 out]
        }
        event "Lateral beam", "save lateral?": Value Change {
          # "3 pt smooth"
          n508 = event-data() -> ()  [unwired: 2 out]
          n509 = Unbundle By Name(w878) -> ("A/D info.# A/D bits"=w896:i16, "A/D info.sample rate MHz"=w917:u16)
          n510 = Unbundle By Name(w878) -> ("Votage scaling.Digitizer (dB)"=w880:sgl)
          n511 = Strip Path(path=w861) -> (stripped path=w899:path, name=w903:string)
          n512 = Unbundle By Name(w878) -> ("Scan Settings.Distance between\nscan lines (um)"=w913:u16)
          n513 = for {
            tunnel: [w955] -> w870 mode=indexing
            tunnel: w890 -> [w954] mode=indexing
            n514 = Absolute Value(x=w954) -> (abs(x)=w953:dbl[])
            n515 = Array Max & Min(array=w953) -> (max value=w955:dbl)  [unwired: 3 out]
          }
          "Peaks" <- w870
          n516 = Absolute Value(x=w890) -> (abs(x)=w872:dbl[][])
          n517 = Concatenate Strings(" lat", ".txt") -> (w902:string)
          n518 = Reciprocal(x=w917) -> (1/x=w916:dbl)
          n519 = Array Max & Min(array=w870) -> (max value=w859:dbl)  [unwired: 3 out]
          n520 = Decrement(x=w896) -> (x-1=w897:i16)
          n521 = Subtract(x=w859, y=20.0) -> ()  [unwired: 1 out]
          n522 = expression code="10**(x/20)"(w880) -> (w892:sgl)
          n523 = call <vilib>:"Peak Detector.vi"("width"="width", "threshold"="Threshold", "X"=w870) -> ("Locations"=w868:dbl[])  [unwired: 4 in, 4 out]
          "Scan Line Peak" <- w868
          n524 = Search and Replace String(input string=w903, search string=".eye", replace string=w902) -> (result string=w900:string)  [unwired: 1 in, 7 out]
          n525 = Power Of 2(x=w897) -> (2^x=w894:dbl)
          n526 = Compound Arithmetic op=MULTIPLY(w877, 0.0005, w916) -> (w915:dbl)
          n527 = Reciprocal(x=w894) -> (1/x=w893:dbl)
          n528 = for {
            tunnel: w890 -> [w949]
            tunnel: [w947] -> w889 mode=indexing
            tunnel: w868 -> [w945] mode=indexing
            tunnel: "Threshold" -> [w946]
            n529 = Index Array(array=w949, index (row)=w945) -> (element=w948:dbl[])  [unwired: 1 in]
            n530 = Threshold 1D Array(2:w946, 3:w948) -> (0:w947:dbl)  [unwired: 1 out]
          }
          "Wire Locations RF pts" <- w889
          n531 = Subtract(x=w889, y=20) -> (x-y=w908:dbl[])
          n532 = for {
            tunnel: w872 -> [w973]
            tunnel: 40 -> [w967]
            tunnel: [w969] -> w895 mode=indexing
            tunnel: w908 -> [w966] mode=indexing
            tunnel: [w968] -> w912
            tunnel: [w964] -> w875
            w971 = 75
            n533 = Array Subset(array=w973, index (col)=w966, length (col)=w967) -> (w965:dbl[][])  [unwired: 2 in]
            n534 = for {
              tunnel: w965 -> [w975] mode=indexing
              tunnel: [w974] -> w956 mode=indexing
              n535 = Array Max & Min(array=w975) -> (max value=w974:dbl)  [unwired: 3 out]
            }
            n536 = Rotate 1D Array(1:w956, 2:1) -> (0:w959:dbl[])
            n537 = Rotate 1D Array(1:w956, 2:-1) -> (0:w958:dbl[])
            n538 = Compound Arithmetic op=ADD(w956, w959, w958) -> (w957:dbl[])
            n539 = Divide(x=w957, y=3) -> (x/y=w961:dbl[])
            n540 = Array Max & Min(array=w956) -> (max index (indices)=w964:i32)  [unwired: 3 out]
            n541 = Subtract(x=w964, y=w971) -> (x-y=w972:i32)
            n542 = Multiply(x=w971, y=2) -> (x*y=w968:i32)
            n543 = Array Subset(array=w961, index=w972, length=w968) -> (w969:dbl[])
          }
          n544 = Multiply(x=w892, y=w893) -> ()  [unwired: 1 out]
          n545 = Build Path(base path=w899, name or relative path=w900) -> (appended path=w898:path)
          n546 = Multiply(x=w915, y=w889) -> (x*y=w919:dbl[])
          n547 = Strip Path(path=w861) -> (name=w860:string)  [unwired: 1 out]
          n548 = for {
            N: w912 -> [_]
            tunnel: w913 -> [w951]
            tunnel: [w952] -> w882 mode=indexing
            i -> [w950]
            n549 = Multiply(x=w951, y=w950) -> (x*y=w952:i32)
          }
          n550 = Add(x=w919, y=w876) -> (x+y=w866:dbl[])
          "Wire Locations mm" <- w866
          n551 = Multiply(x=1, y=w895) -> (x*y=w874:dbl[][])
          n552 = Index Array(array=w866) -> (element=w865:dbl)  [unwired: 1 in]
          n553 = Index Array(array=w868) -> (element=w867:dbl)  [unwired: 1 in]
          n554 = Divide(x=w882, y=1000) -> (x/y=w873:dbl[])
          n555 = Build Array (concatenate)(w873, w874) -> (w911:dbl[][])
          "lat beams" <- w911
          n556 = Build Array (concatenate)(w875, w866) -> (w910:dbl[])
          n557 = Transpose 2D Array(2D array=w911) -> (transposed array=w909:dbl[][])
          n558 = for {
            tunnel: w873 -> [w932]
            tunnel: w874 -> [w931] mode=indexing
            tunnel: [w928] -> w858 mode=indexing
            n559 = call "BeamWidthCalc.vi"("Not dB?"=TRUE ("Is dB?"), "dB width pt"=-6.0, "y values"=w931, "x values"=w932) -> ("Output variables"=w929:T34)  [unwired: 5 in, 2 out]
            n560 = Unbundle By Name(w929) -> ("bandwidth"=w928:sgl)
          }
          "Beamwidths" <- w858
          n561 = Build Array (concatenate)(w910, w909) -> (w906:dbl[][])
          n562 = for {
            tunnel: w868 -> [w941] mode=indexing
            tunnel: w890 -> [w942]
            tunnel: w889 -> [w939] mode=indexing
            tunnel: [w935] -> w887 mode=indexing
            tunnel: 25 ("length") -> [w938]
            tunnel: 50 ("length") -> [w936]
            n563 = Subtract(x=w939, y=w938) -> (x-y=w937:dbl)
            n564 = Array Subset(array=w942, index (row)=w941, length (row)=1 ("length"), index (col)=w937, length (col)=w936) -> (w934:dbl[][])
            n565 = Absolute Value(x=w934) -> (abs(x)=w933:dbl[][])
            n566 = Array Max & Min(array=w933) -> (max value=w935:dbl)  [unwired: 3 out]
          }
          n567 = case shown="True" "save lateral?" {
            tunnel: w906 -> [_ w943]
            tunnel: w898 -> [_ w944]
            frame False {
            }
            frame True {
              n568 = call-poly <vilib>:"Write Delimited Spreadsheet.vi"("file path (dialog if empty)"=w944, "2D data"=w943) -> ()  [unwired: 12 in, 2 out]
            }
          }
          n569 = local read "RMS noise"() -> (w886:dbl)
          n570 = Divide(x=w887, y=w886) -> (x/y=w888:dbl[])
          n571 = Index Array(array=w858) -> (element=w857:sgl)  [unwired: 1 in]
          n572 = Build Array(w859, w865, w867, w857) -> (w864:dbl[])
          n573 = case shown="True" "Boolean" {
            tunnel: w864 -> [_ w923]
            tunnel: path "C:/Users/jketterling/Desktop/New Text Document.txt" ("file path (dialog if empty)") -> [_ w925]
            tunnel: w860 -> [_ w924]
            frame False {
            }
            frame True {
              n574 = Number To Fractional String(number=w923) -> (F-format string=w922:string[])  [unwired: 3 in]
              n575 = Build Array (concatenate)(w924, w922) -> (w921:string[])
              n576 = call-poly <vilib>:"Write Delimited Spreadsheet.vi"("file path (dialog if empty)"=w925, "1D data"=w921, "append to file? (new file:F)"=TRUE) -> ()  [unwired: 11 in, 2 out]
            }
          }
          n577 = expression code="20*log(x)"(w888) -> (w885:dbl[])
          n578 = local write "SNRs"(w885) -> ()
        }
        event "Center Line SNR": Value Change {
          n579 = event-data() -> ()  [unwired: 7 out]
          n580 = Index Array(array=w984, index (row)="Center index") -> (element=w982:dbl[])  [unwired: 1 in]
          n581 = Array Size(array=w982) -> (size(s)=w988:i32)
          n582 = Divide(x=w988, y="Wires") -> (x/y=w986:dbl)
          n583 = Divide(x=w986, y=2.0) -> (x/y=w985:dbl)
          n584 = for {
            N: "Wires" -> [_]
            tunnel: w986 -> [w993]
            tunnel: w985 -> [w995]
            tunnel: w982 -> [w994]
            tunnel: [w990] -> w979 mode=indexing
            i -> [w996]
            n585 = Multiply(x=w993, y=w996) -> (x*y=w989:dbl)
            n586 = Add(x=w995, y=w989) -> ()  [unwired: 1 out]
            n587 = Array Subset(array=w994, index=w989, length=w993) -> (w992:dbl[])
            n588 = Absolute Value(x=w992) -> (abs(x)=w991:dbl[])
            n589 = Array Max & Min(array=w991) -> (max value=w990:dbl)  [unwired: 3 out]
          }
          n590 = local read "RMS noise"() -> (w978:dbl)
          n591 = Divide(x=w979, y=w978) -> (x/y=w980:dbl[])
          n592 = expression code="20*log(x)"(w980) -> (→"SNRs":dbl[])
        }
        event "Spectrum?": Value Change {
          n593 = event-data() -> ()  [unwired: 2 out]
          n594 = Unbundle By Name(w999) -> ("A/D info.sample rate MHz"=w998:u16)
          n595 = Reciprocal(x=w998) -> (1/x=w1034:dbl)
          n596 = local read "blue win"() -> (w1022:dbl[])
          n597 = Initialize Array(0, 100) -> (w1030:i32[])
          n598 = Build Array (concatenate)(w1030, w1022) -> (w1000:dbl[])
          n599 = expression code="2**(x+2)"("STFT size") -> (w1001:u16)
          n600 = Divide(x=w998, y=w1001) -> (x/y=w1028:dbl)
          n601 = Array Size(array=w1000) -> (size(s)=w1023:i32)
          n602 = Bundle("step size"="step size", "STFT size"=w1001) -> (w1009:cluster{"step size":i32, "STFT size":u16})  [unwired: 1 in]
          n603 = Bundle("Window"="Window", "window pts"="window pts") -> (w1006:cluster{"Window":u32, "window pts":i32})  [unwired: 1 in]
          n604 = Divide(x=w1023, y="step size") -> (x/y=w1017:dbl)
          n605 = Multiply(x="step size", y=w1034) -> (x*y=w1033:dbl)
          n606 = Multiply(x=w1034, y="window pts") -> (x*y=→"Time step (mics)":dbl)
          n607 = Add(x=13, y=w1017) -> (x+y=w1016:dbl)
          n608 = call <vilib>:"STFT Spectrograms.vi"("energy conservation?"=FALSE, "window info"=w1006, "time-freq sampling info"=w1009, "X"=w1000) -> ("STFT Spectrogram {X}"=w1003:dbl[][])  [unwired: 6 in, 1 out]
          n609 = property on="Spectro fig" class="IntGraph (strict)"("X Scale.Offset and Multiplier:Multiplier"=w1033, "Y Scale.Offset and Multiplier:Multiplier"=w1028) -> ()  [unwired: 2 in, 2 out]
          n610 = Divide(x=20, y=w1028) -> (x/y=w1025:dbl)
          n611 = Divide(x=40, y=w1028) -> (x/y=w1024:dbl)
          n612 = Array Subset(array=w1003, length (row)=w1016) -> (w1005:dbl[][])  [unwired: 3 in]
          n613 = expression code="10*log(x+1E-7)"(w1005) -> (w1019:dbl[][])
          n614 = Array Max & Min(array=w1019) -> (max value=w1011:dbl)  [unwired: 3 out]
          "max value" <- w1011
          n615 = Index Array(array=w1019, index (col)=w1025) -> (element=w1015:dbl[])  [unwired: 1 in]
          "Waveform Graph" <- w1015
          n616 = Index Array(array=w1019, index (col)=w1024) -> (element=w1014:dbl[])  [unwired: 1 in]
          "Waveform Graph 2" <- w1014
          n617 = Subtract(x=w1019, y="Shift") -> (x-y=w1013:dbl[][])
          n618 = Subtract(x=w1013, y=w1011) -> (x-y=→"Spectro fig":dbl[][])
          n619 = call <vilib>:"Pulse Parameters.vi"("X"=w1015) -> ("top"=→"mean":dbl)  [unwired: 14 out]
          n620 = call <vilib>:"Pulse Parameters.vi"("X"=w1014) -> ("top"=→"mean 2":dbl)  [unwired: 14 out]
        }
        event "Spectro BMP": Value Change {
          # "Change to 8-bit"
          n621 = event-data() -> ()  [unwired: 7 out]
          n622 = invoke on="Spectro fig" class="IntGraph (strict)" method="Get Image"("image depth"=24) -> ("image data"=w1037:T20)  [unwired: 5 in, 5 out]
          n623 = call <vilib>:"Write BMP File.vi"("image data"=w1037) -> ()  [unwired: 2 in, 9 out]
        }
        event "Histo": Value Change {
          n624 = event-data() -> ()  [unwired: 2 out]
          n625 = Strip Path(path=w1045) -> (stripped path=w1040:path, name=w1048:string)
          n626 = Match Pattern(string=w1048, regular expression="....eye") -> (before substring=w1050:string, match substring=w1042:string)  [unwired: 3 out]
          n627 = Concatenate Strings(w1050, ".txt" ("regular expression")) -> (w1051:string)
          n628 = Match Pattern(string=w1042, regular expression=".eye") -> (before substring=w1044:string)  [unwired: 4 out]
          n629 = Build Path(base path=w1040, name or relative path=w1051) -> (appended path=w1047:path)
          n630 = Decimal String To Number(string=w1044) -> (number=w1041:i32)  [unwired: 3 out]
          n631 = call-poly <vilib>:"Read Delimited Spreadsheet.vi"("file path (dialog if empty)"=w1047) -> ("all rows"=w1046:i64[][])  [unwired: 9 in, 5 out]
          n632 = call "CAHistogram.vi"("Peak File?"=TRUE, "index"=w1041, "all rows"=w1046) -> ("Histogram"=→"XY Graph":T7)  [unwired: 1 in, 1 out]
        }
        event "Contrast Spec": Value Change {
          n633 = event-data() -> ()  [unwired: 3 out]
          n634 = Unbundle By Name(w1056) -> ("Therapy Parameters.Therapy amplitude (mV)"=→"Therapy amplitude (mV)":sgl)
          n635 = call "CA Spectra.vi"("Header In"=w1056, "Data in"=w1059, "2nd freq"=20, "sub thresh"="sub thresh") -> ("Windowed RF traces"=→"time trace":dbl[][], "ratio histo"=→"histogram":T7, "Spectra"=→"Sepctra":cluster{i32, "df":dbl, dbl[][]}, "output params"=w1058:T35, "Scatter"=→"?":cluster{dbl[], "Best Linear Fit":dbl[]}[])  [unwired: 5 in, 6 out]
          n636 = Unbundle By Name(w1058) -> ("Hit frac"=→"Hit frac":dbl)
        }
        event "Contrast Batch": Value Change {
          n637 = event-data() -> ()  [unwired: 2 out]
          n638 = Strip Path(path=w1069) -> (stripped path=w1068:path)  [unwired: 1 out]
          n639 = call "CA Batch.vi"("Select directory with EYE files"=w1068) -> ()  [unwired: 6 out]
        }
        event "Match Filter": Value Change {
          n640 = event-data() -> ()  [unwired: 7 out]
          n641 = Unbundle By Name(w1071) -> ("Compression Parameters.duration"=w1077:sgl, "Compression Parameters.% taper"=w1082:sgl, "Compression Parameters.F1 (MHz)"=w1078:sgl, "Compression Parameters.F2 (MHz)"=w1079:sgl)
          n642 = Unbundle By Name(w1071) -> ("A/D info.sample rate MHz"=w1086:u16)
          n643 = Multiply(x=w1086, y=w1077) -> (x*y=w1081:sgl)
          n644 = Reciprocal(x=w1086) -> (1/x=w1080:dbl)
          n645 = call "Tukey.vi"("f2 (MHz)"=w1079, "f1 (MHz)"=w1078, "Samp Rate (mics)"=w1080, "Pts"=w1081, "Tukey"=w1082) -> ("Tukey Chirp"=w1075:dbl[])  [unwired: 2 in, 4 out]
          n646 = call-poly <vilib>:"Chebyshev Window.vi"("lobe ratio (dB)"=90.0, "X"=w1075) -> ()  [unwired: 10 out]
          n647 = Reverse 1D Array(array=w1075) -> (reversed array=w1076:dbl[])
          n648 = call "Compress Chirp.vi"("Chirp"=w1076, "Array In"=w1085) -> ("Array Out"=w1073:dbl[][])
          "Chirp Temp" <- w1073
          n649 = call <vilib>:"Quick Scale 2D.vi"("X"=w1073) -> ("Yij=Xij/Max|X|"=w1074:dbl[][])  [unwired: 2 out]
          n650 = expression code="20*log(abs(x))"(w1074) -> (w1072:dbl[][])
          n651 = Transpose 2D Array(2D array=w1072) -> (transposed array=→"Match Data":dbl[][])
        }
        event "Save Chirp": Value Change {
          w1098 = 16
          n652 = event-data() -> ()  [unwired: 7 out]
          n653 = Bundle By Name(cluster=w1099, "A/D info.# A/D bits"=w1098, "A/D info.# bytes per A/D"=2) -> (w1088:T17)
          n654 = Strip Path(path=w1095) -> (stripped path=w1091:path, name=w1094:string)
          n655 = Concatenate Strings("COM" ("string"), w1094) -> (w1092:string)
          n656 = Build Path(base path=w1091, name or relative path=w1092) -> (appended path=w1089:path)
          n657 = Decrement(x=w1098) -> (x-1=w1103:i32)
          n658 = local read "Chirp Temp"() -> (w1096:dbl[][])
          n659 = Power Of 2(x=w1103) -> (2^x=w1102:dbl)
          n660 = Decrement(x=w1102) -> (x-1=w1101:dbl)
          n661 = call-poly <vilib>:"Quick Scale.vi"("X"=w1096) -> ("Yij=Xij/Max|X|"=w1100:dbl[][])  [unwired: 2 out]
          n662 = Multiply(x=w1101, y=w1100) -> (x*y=w1090:dbl[][])
          n663 = call "SaveDataFast.vi"("Header In"=w1088, "Data Array"=w1090, "File Name and Path"=w1089) -> ()  [unwired: 8 in, 1 out]
        }
        event "Retro Parse": Value Change {
          n664 = event-data() -> ()  [unwired: 2 out]
          n665 = Strip Path(path=w1106) -> (stripped path=w1105:path)  [unwired: 1 out]
          n666 = call "RetroParse.vi"("Choose Directory"=w1105) -> ()  [unwired: 11 out]
        }
        event "Heart Trig": Value Change {
          w1115 = 1000
          n667 = event-data() -> ()  [unwired: 2 out]
          n668 = Initialize Array(0.0 ("element"), w1115) -> (w1116:dbl[])
          n669 = for {
            tunnel: "Edge Thresh" -> [w1150]
            tunnel: w1109 -> [w1148] mode=indexing
            tunnel: [w1158] -> w1118 mode=indexing
            tunnel: [w1145] -> w1120 mode=indexing
            shift-right: [w1126] -> _
            shift-left: w1116 -> [w1157]
            shift-left: w1116 -> [w1156]
            shift-left: w1116 -> [w1154]
            tunnel: [w1126] -> w1123 mode=indexing
            tunnel: "initial Skip index" -> [w1146]
            shift-left: w1116 -> [w1138]
            tunnel: w1115 -> [w1141]
            shift-right: [w1130] -> _
            shift-left: FALSE -> [w1131]
            i -> [w1139]
            n670 = call <vilib>:"Fast Hilbert Transform.vi"("X"=w1148) -> ("Hilbert{X}"=w1152:dbl[])  [unwired: 1 out]
            n671 = case shown="4, Default" w1139 {
              selector: w1139 -> [w1164 w1166 w1168 w1170 _]
              tunnel: [w1163 w1165 w1167 w1169 5] -> w1151
              frame 0 {
                n672 = Increment(x=w1164) -> (x+1=w1163:i32)
              }
              frame 1 {
                n673 = Increment(x=w1166) -> (x+1=w1165:i32)
              }
              frame 2 {
                n674 = Increment(x=w1168) -> (x+1=w1167:i32)
              }
              frame 3 {
                n675 = Increment(x=w1170) -> (x+1=w1169:i32)
              }
              frame 4, Default {
              }
            }
            n676 = Re/Im To Complex(1:w1152, 2:w1148) -> (0:w1153:cdb[])
            n677 = Absolute Value(x=w1153) -> (abs(x)=w1147:dbl[])
            n678 = Array Subset(array=w1147, index=w1146, length=w1141) -> (w1144:dbl[])
            n679 = call <vilib>:"Median Filter.vi"("right rank"="AS Med Fil", "left rank"="AS Med Fil", "X"=w1144) -> ("Filtered X"=w1127:dbl[])  [unwired: 8 out]
            n680 = Compound Arithmetic op=ADD(w1157, w1156, w1154, w1138, w1127) -> (w1155:dbl[])
            n681 = Divide(x=w1155, y=w1151) -> (x/y=w1126:dbl[])
            n682 = Threshold 1D Array(2:w1150, 3:w1126) -> (0:w1129:dbl)  [unwired: 1 out]
            n683 = Equal To 0?(x=w1139) -> (x = 0?=w1137:bool)
            n684 = call <vilib>:"Derivative x(t) PtByPt.vi"("initialize"=w1137, "initial condition"=w1129, "x"=w1129) -> ("dx/dt"=w1142:dbl)  [unwired: 1 in, 1 out]
            n685 = call <vilib>:"Median PtByPt.vi"("initialize"=w1137, "sample length"="Thresh Median Lngth", "x"=w1142) -> ("median"=w1134:dbl)  [unwired: 2 out]
            n686 = expression code="x+2"("Thresh Median Lngth") -> (w1140:i32)
            n687 = Less?(x=w1134, y="neg cross") -> (x < y?=w1132:bool)
            n688 = call <vilib>:"Zero Crossing PtByPt.vi"("initialize"=w1137, "direction"="direction", "input data point"=w1134) -> ("crossing"=w1136:bool)
            n689 = Greater Or Equal?(x=w1139, y=w1140) -> (x >= y?=w1149:bool)
            n690 = Or(x=w1132, y=w1131) -> (x .or. y?=w1130:bool)
            n691 = case shown="True" w1149 {
              tunnel: w1136 -> [_ w1160]
              tunnel: [_ w1159] -> w1158
              tunnel: [_ w1162] -> w1145
              tunnel: w1134 -> [_ w1162]
              tunnel: w1130 -> [_ w1161]
              frame False {
              }
              frame True {
                n692 = And(x=w1160, y=w1161) -> (x .and. y?=w1159:bool)
                "Smooth dat" <- w1162
              }
            }
          }
          "Avg Env image" <- w1123
          n693 = call "SmoothSurface.vi"("Bit Depth"=w1108, "Eye in"=w1109) -> ("Smooth out"=w1112:i16[][])  [unwired: 9 out]
          n694 = Transpose 2D Array(2D array=w1112) -> (transposed array=w1111:i16[][])
          n695 = call "LogScaleImage.vi"("A/D bits"=u16 8, "input array"=w1111) -> ()  [unwired: 2 out]
          n696 = Boolean To (0,1)(Boolean=w1118) -> (0, 1=w1119:i16[])
          n697 = Array Max & Min(array=w1120) -> (max value=w1121:dbl)  [unwired: 3 out]
          n698 = Multiply(x=w1119, y=w1121) -> (x*y=w1124:dbl[])
          n699 = Build Array(w1120, w1124) -> (→"Overlay":dbl[][])
        }
        event "Ebedded EKG": Value Change {
          n700 = event-data() -> ()  [unwired: 2 out]
          n701 = case shown="0, Default" "EKG Gate" {
            tunnel: w1176 -> [w1190 w1197]
            tunnel: w1173 -> [w1177 w1191]
            tunnel: [w1178 w1198] -> w1174
            frame 0, Default {
              n702 = Open/Create/Replace File(file path (use dialog)=w1190) -> (refnum out=w1188:refnum<file>, error out=w1189:errorcluster)  [unwired: 1 in, 5 out]
              n703 = Unbundle By Name(w1177) -> ("A/D info.# lines per scan"=w1184:u16)
              n704 = Set File Position(offset (in bytes) (0)=i64 1024, refnum=w1188, error in=w1189) -> (refnum out=w1187:refnum<file>, error out=w1186:errorcluster)  [unwired: 1 out]
              n705 = Read from Binary File(5:i16 0, 8:w1186, 9:T16."little-endian" ("byte order (0:big-endian, network order)"), 10:w1184, 11:w1187) -> (0:w1182:errorcluster, 2:w1179:i16[], 3:w1181:refnum<file>)  [unwired: 2 out]
              n706 = Close File(refnum=w1181, error in=w1182) -> ()  [unwired: 2 out]
              n707 = Build Array(w1179) -> (w1178:i16[][])
            }
            frame 1 {
              n708 = Strip Path(path=w1197) -> (stripped path=w1196:path, name=w1207:string)
              n709 = Unbundle By Name(w1191) -> ("Scan Settings.prf (kHz)"=w1214:sgl)
              n710 = Unbundle By Name(w1191) -> ("A/D info.# lines per scan"=w1215:u16)
              n711 = Search and Replace String(input string=w1207, search string="eye", replace string="IQ") -> (result string=w1195:string)  [unwired: 1 in, 7 out]
              n712 = Build Path(base path=w1196, name or relative path=w1195) -> (appended path=w1194:path)
              n713 = Reciprocal(x=w1214) -> (1/x=w1209:sgl)
              n714 = Open/Create/Replace File(file path (use dialog)=w1194) -> (refnum out=w1193:refnum<file>, error out=w1192:errorcluster)  [unwired: 1 in, 5 out]
              n715 = Compound Arithmetic op=MULTIPLY(24, w1209, w1215) -> (w1201:sgl)
              n716 = Multiply(x=w1201, y=2) -> (x*y=w1203:sgl)
              n717 = Read from Binary File(5:i16 0, 8:w1192, 9:T16."little-endian" ("byte order (0:big-endian, network order)"), 10:w1203, 11:w1193) -> (0:w1212:errorcluster, 2:w1204:i16[], 3:w1211:refnum<file>)  [unwired: 2 out]
              n718 = Close File(refnum=w1211, error in=w1212) -> ()  [unwired: 2 out]
              n719 = Split 1D Array(array=w1204, index=w1201) -> (first subarray=w1200:i16[], second subarray=w1199:i16[])
              n720 = Build Array(w1200, w1199) -> (w1198:i16[][])
            }
          }
          "EKG" <- w1174
        }
        event "Type of Mean", "Filter Prams": Value Change {
          n721 = event-data() -> ()  [unwired: 7 out]
        }
        event "Sound Speed": Value Change {
          n722 = event-data() -> ()  [unwired: 7 out]
        }
        event "Keeper?": Value Change {
          # "This will add a sring to previsiously scanned position in header. Used now to mark floaters."
          n723 = event-data() -> ()  [unwired: 3 out]
          n724 = Bundle By Name(cluster=w1232, "Patient Info.previously\nscanned"="previously\nscanned") -> (w1230:T17)
          n725 = call "MakeHeader.vi"("Header In"=w1230) -> ("Header String"=w1223:string)  [unwired: 6 out]
          n726 = Open/Create/Replace File(file path (use dialog)=w1229) -> (refnum out=w1228:refnum<file>, error out=w1227:errorcluster)  [unwired: 5 in, 1 out]
          n727 = Set File Position(refnum=w1228, error in=w1227) -> (refnum out=w1224:refnum<file>)  [unwired: 2 in, 1 out]
          n728 = Write to Binary File(file (use dialog)=w1224, data=w1223, 5:FALSE ("prepend array or string size? (T)")) -> (refnum out=w1221:refnum<file>, error out=w1222:errorcluster)  [unwired: 3 in, 1 out]
          n729 = Close File(refnum=w1221, error in=w1222) -> ()  [unwired: 2 out]
        }
        event "left rank", "medians": Value Change {
          # "Was for median filter testing in floater routine."
          n730 = event-data() -> ()  [unwired: 7 out]
        }
        event "Log": Value Change {
          # "This will log ROI values in floater routine to a file. Can also use auto step through."
          n731 = event-data() -> ()  [unwired: 7 out]
        }
        event "Log noise window": Value Change {
          # "THis will save ROI positions within the eye file. Used for noise ROI but could be anything."
          # "Take window"
          # "Scale accordingly"
          n732 = event-data() -> ()  [unwired: 5 out]
          n733 = property on="Raw data" class="IntGraph (strict)"() -> ("XScale.Offset"=w1264:dbl, "XScale.Multiplier"=w1263:dbl, "YScale.Multiplier"=w1262:dbl)  [unwired: 2 in, 2 out]
          n734 = property on="Raw data" class="IntGraph (strict)"("Active Cursor"=u32 0 ("Write Attribute"), "Active Cursor"=u32 1 ("Write Attribute")) -> ("Cursor.Cursor X"=w1261:dbl, "Cursor.Cursor Y"=w1257:dbl, "Cursor.Cursor X"=w1260:dbl, "Cursor.Cursor Y"=w1256:dbl)  [unwired: 2 in, 2 out]
          n735 = Subtract(x=w1260, y=w1264) -> (x-y=w1266:dbl)
          n736 = Subtract(x=w1261, y=w1264) -> (x-y=w1267:dbl)
          n737 = Divide(x=w1267, y=w1263) -> (x/y=w1255:dbl)
          n738 = Divide(x=w1257, y=w1262) -> (x/y=w1268:dbl)
          n739 = Divide(x=w1266, y=w1263) -> (x/y=w1265:dbl)
          n740 = Divide(x=w1256, y=w1262) -> (x/y=w1242:dbl)
          n741 = Subtract(x=w1265, y=w1255) -> (x-y=w1254:dbl)
          n742 = Subtract(x=w1268, y=w1242) -> (x-y=w1241:dbl)
          n743 = Build Array(w1242, w1241, w1255, w1254) -> (w1253:dbl[])
          n744 = To Unsigned Word Integer(number=w1253) -> (unsigned 16bit integer=w1245:u16[])
          n745 = Bundle By Name(cluster=w1246, "ROI Box"=w1245) -> (w1252:T17)
          n746 = call "MakeHeader.vi"("Header In"=w1252) -> ("Header String"=w1250:string)  [unwired: 6 out]
          n747 = Open/Create/Replace File(file path (use dialog)=w1244) -> (refnum out=w1249:refnum<file>, error out=w1248:errorcluster)  [unwired: 5 in, 1 out]
          n748 = Set File Position(refnum=w1249, error in=w1248) -> (refnum out=w1247:refnum<file>, error out=w1240:errorcluster)  [unwired: 2 in]
          n749 = Write to Binary File(file (use dialog)=w1247, data=w1250, error in=w1240, 5:FALSE ("prepend array or string size? (T)")) -> (refnum out=w1251:refnum<file>, error out=w1239:errorcluster)  [unwired: 2 in, 1 out]
          n750 = Close File(refnum=w1251, error in=w1239) -> ()  [unwired: 2 out]
        }
      }
      n751 = Or(x=w71, y="ExitSendCmd") -> (x .or. y?=w70:bool)
    }
  }
